vi "Strategy 5_Autotuning PID_With GUI - Copy (3).vi"() -> ()   [LabVIEW 2018]
doc: "This example demonstrates how to use the PID Design function to obtain PID parameters based on measured process."
uses:
  <vilib>/DAQmx/write.llb/DAQmx Write (Digital 1D Bool 1Chan 1Samp).vi
  <vilib>/Instr/_visa.llb/VISA Configure Serial Port (Instr).vi
  <vilib>/DAQmx/create/channels.llb/DAQmx Create Channel (DO-Digital Output).vi
  <vilib>/DAQmx/miscellaneous.llb/DAQmx Fill In Error Info.vi
  <vilib>/addons/control/pid/pid.llb/PID Advanced (DBL).vi
  <vilib>/addons/control/pid/autopid.llb/PID Autotuning Design (Ziegler-Nichols).vi
  <vilib>/addons/control/pid/autopid.llb/PID Autotuning Design (Cohen-Coon).vi
  <vilib>/addons/control/pid/autopid.llb/PID Autotuning Design (Chien-Hrones-Reswick).vi
  <vilib>/addons/control/pid/autopid.llb/PID Autotuning Design (Internal Model Control).vi
  <vilib>/addons/control/pid/NI_PID_autopid.lvlib
  <vilib>/addons/control/pid/NI_PID_pid.lvlib
  <vilib>/ptbypt/NI_PtbyPt.lvlib
panel:
  out "?":bool
  in  "Muscle Control":T1(tab)=enum."M-11"
  out "Tuned PID gains 12":T2={"proportional gain (Kc)"=1.9838195929127882, "integral time (Ti, min)"=0.01995856284686879, "derivative time (Td, min)"=0.0} {"derivative time (Td, min)" format="%#.6g"; "integral time (Ti, min)" format="%#.6g"; "proportional gain (Kc)" format="%#.6g"}
  in  "Accept gain 12":bool
  in  "Control 12":T3(tab)
  in  "Ziegler-Nichols speed 12":u16(ring) items=["Fast", "Normal", "Slow"]
  in  "Tuning specifications 12":u16(ring) items=["Regulator - 0 %", "Regulator -  20%", "Servo - 0%", "Servo - 20%"]
  in  "Multiplicative factor 12":dbl(slide)=1.0 scale=0.01..100.0
  in  "Type of controller 12":u16(ring)=2 items=["P", "PI", "PID"]
  in  "Stop 12":bool
  in  "PID Gains 12":T2={"proportional gain (Kc)"=0.1625, "integral time (Ti, min)"=1.25, "derivative time (Td, min)"=0.0} {"derivative time (Td, min)" format="%#.6g"; "integral time (Ti, min)" format="%#.6g"; "proportional gain (Kc)" format="%#.6g"}
  in  "Autotune 12":bool
  in  "Reinitialize 12":bool
  in  "Excitation 12":dbl=0.5 format="%.2f"
  in  "Automatic 12":bool=TRUE
  in  "MV: 12":dbl(slide)=20.39115328927357 scale=-100.0..100.0
  in  "Set Point 12":dbl(slide) scale=0.0..30.0
  out "PWM Output 12":bool
  out "Real time Data 12":dbl[][](graph)
  in  "Median sample length 21":i32=100
  in  "INLET 1 ON/OFF 3":bool=TRUE
  out "Tuned PID gains 11":T2={"proportional gain (Kc)"=1.9838195929127882, "integral time (Ti, min)"=0.01995856284686879, "derivative time (Td, min)"=0.0} {"derivative time (Td, min)" format="%#.6g"; "integral time (Ti, min)" format="%#.6g"; "proportional gain (Kc)" format="%#.6g"}
  in  "Accept gain 11":bool
  in  "Control 11":T3(tab)
  in  "Ziegler-Nichols speed 11":u16(ring) items=["Fast", "Normal", "Slow"]
  in  "Tuning specifications 11":u16(ring) items=["Regulator - 0 %", "Regulator -  20%", "Servo - 0%", "Servo - 20%"]
  in  "Multiplicative factor 11":dbl(slide)=1.0 scale=0.01..100.0
  in  "Type of controller 11":u16(ring)=2 items=["P", "PI", "PID"]
  in  "Excitation 11":dbl=0.5 format="%.2f"
  in  "Stop 11":bool
  in  "PID Gains 11":T2={"proportional gain (Kc)"=0.1625, "integral time (Ti, min)"=1.25, "derivative time (Td, min)"=0.0} {"derivative time (Td, min)" format="%#.6g"; "integral time (Ti, min)" format="%#.6g"; "proportional gain (Kc)" format="%#.6g"}
  in  "Autotune 11":bool
  in  "Reinitialize 11":bool
  in  "Automatic 11":bool=TRUE
  in  "MV: 11":dbl(slide)=20.39115328927357 scale=-100.0..100.0
  in  "Set Point 11":dbl(slide) scale=0.0..30.0
  out "PWM Output 11":bool
  out "Real time Data 11":dbl[][](graph)
  in  "Median sample length 20":i32=100
  in  "INLET 5 ON/OFF 3":bool=TRUE
  out "Tuned PID gains 10":T2={"proportional gain (Kc)"=1.9838195929127882, "integral time (Ti, min)"=0.01995856284686879, "derivative time (Td, min)"=0.0} {"derivative time (Td, min)" format="%#.6g"; "integral time (Ti, min)" format="%#.6g"; "proportional gain (Kc)" format="%#.6g"}
  in  "Accept gain 10":bool
  in  "Control 10":T3(tab)
  in  "Ziegler-Nichols speed 10":u16(ring) items=["Fast", "Normal", "Slow"]
  in  "Tuning specifications 10":u16(ring) items=["Regulator - 0 %", "Regulator -  20%", "Servo - 0%", "Servo - 20%"]
  in  "Multiplicative factor 10":dbl(slide)=1.0 scale=0.01..100.0
  in  "Type of controller 10":u16(ring)=2 items=["P", "PI", "PID"]
  in  "Stop 10":bool
  in  "PID Gains 10":T2={"proportional gain (Kc)"=0.1625, "integral time (Ti, min)"=1.25, "derivative time (Td, min)"=0.0} {"derivative time (Td, min)" format="%#.6g"; "integral time (Ti, min)" format="%#.6g"; "proportional gain (Kc)" format="%#.6g"}
  in  "Autotune 10":bool
  in  "Reinitialize 10":bool
  in  "Excitation 10":dbl=0.5 format="%.2f"
  in  "Automatic 10":bool=TRUE
  in  "MV: 10":dbl(slide)=20.39115328927357 scale=-100.0..100.0
  in  "Set Point 10":dbl(slide) scale=0.0..30.0
  out "PWM Output 10":bool
  out "Real time Data 10":dbl[][](graph)
  in  "Median sample length 19":i32=100
  in  "INLET 3 ON/OFF 3":bool=TRUE
  out "Tuned PID gains 9":T2={"proportional gain (Kc)"=1.9838195929127882, "integral time (Ti, min)"=0.01995856284686879, "derivative time (Td, min)"=0.0} {"derivative time (Td, min)" format="%#.6g"; "integral time (Ti, min)" format="%#.6g"; "proportional gain (Kc)" format="%#.6g"}
  in  "Accept gain 9":bool
  in  "Type of controller 9":u16(ring)=2 items=["P", "PI", "PID"]
  in  "Excitation 9":dbl=0.5 format="%.2f"
  in  "Control 9":T3(tab)
  in  "Ziegler-Nichols speed 9":u16(ring) items=["Fast", "Normal", "Slow"]
  in  "Tuning specifications 9":u16(ring) items=["Regulator - 0 %", "Regulator -  20%", "Servo - 0%", "Servo - 20%"]
  in  "Multiplicative factor 9":dbl(slide)=1.0 scale=0.01..100.0
  in  "Stop 9":bool
  in  "PID Gains 9":T2={"proportional gain (Kc)"=0.1625, "integral time (Ti, min)"=1.25, "derivative time (Td, min)"=0.0} {"derivative time (Td, min)" format="%#.6g"; "integral time (Ti, min)" format="%#.6g"; "proportional gain (Kc)" format="%#.6g"}
  in  "Autotune 9":bool
  in  "Reinitialize 9":bool
  in  "Automatic 9":bool=TRUE
  in  "MV: 9":dbl(slide)=20.39115328927357 scale=-100.0..100.0
  in  "Set Point 9":dbl(slide) scale=0.0..30.0
  out "PWM Output 9":bool
  out "Real time Data 9":dbl[][](graph)
  in  "Median sample length 18":i32=100
  in  "INLET 10 ON/OFF 2":bool=TRUE
  out "Tuned PID gains 8":T2={"proportional gain (Kc)"=1.9838195929127882, "integral time (Ti, min)"=0.01995856284686879, "derivative time (Td, min)"=0.0} {"derivative time (Td, min)" format="%#.6g"; "integral time (Ti, min)" format="%#.6g"; "proportional gain (Kc)" format="%#.6g"}
  in  "Accept gain 8":bool
  in  "Control 8":T3(tab)
  in  "Ziegler-Nichols speed 8":u16(ring) items=["Fast", "Normal", "Slow"]
  in  "Tuning specifications 8":u16(ring) items=["Regulator - 0 %", "Regulator -  20%", "Servo - 0%", "Servo - 20%"]
  in  "Multiplicative factor 8":dbl(slide)=1.0 scale=0.01..100.0
  in  "Type of controller 8":u16(ring)=2 items=["P", "PI", "PID"]
  in  "Stop 8":bool
  in  "PID Gains 8":T2={"proportional gain (Kc)"=0.1625, "integral time (Ti, min)"=1.25, "derivative time (Td, min)"=0.0} {"derivative time (Td, min)" format="%#.6g"; "integral time (Ti, min)" format="%#.6g"; "proportional gain (Kc)" format="%#.6g"}
  in  "Autotune 8":bool
  in  "Reinitialize 8":bool
  in  "Excitation 8":dbl=0.5 format="%.2f"
  in  "Automatic 8":bool=TRUE
  in  "MV: 8":dbl(slide)=20.39115328927357 scale=-100.0..100.0
  in  "Set Point 8":dbl(slide) scale=0.0..30.0
  out "PWM Output 8":bool
  out "Real time Data 8":dbl[][](graph)
  in  "Median sample length 17":i32=100
  in  "INLET 2 ON/OFF 2":bool=TRUE
  out "Tuned PID gains 7":T2={"proportional gain (Kc)"=1.9838195929127882, "integral time (Ti, min)"=0.01995856284686879, "derivative time (Td, min)"=0.0} {"derivative time (Td, min)" format="%#.6g"; "integral time (Ti, min)" format="%#.6g"; "proportional gain (Kc)" format="%#.6g"}
  in  "Accept gain 7":bool
  in  "Control 7":T3(tab)
  in  "Ziegler-Nichols speed 7":u16(ring) items=["Fast", "Normal", "Slow"]
  in  "Tuning specifications 7":u16(ring) items=["Regulator - 0 %", "Regulator -  20%", "Servo - 0%", "Servo - 20%"]
  in  "Multiplicative factor 7":dbl(slide)=1.0 scale=0.01..100.0
  in  "Type of controller 7":u16(ring)=2 items=["P", "PI", "PID"]
  in  "Stop 7":bool
  in  "PID Gains 7":T2={"proportional gain (Kc)"=0.1625, "integral time (Ti, min)"=1.25, "derivative time (Td, min)"=0.0} {"derivative time (Td, min)" format="%#.6g"; "integral time (Ti, min)" format="%#.6g"; "proportional gain (Kc)" format="%#.6g"}
  in  "Autotune 7":bool
  in  "Reinitialize 7":bool
  in  "Excitation 7":dbl=0.5 format="%.2f"
  in  "Automatic 7":bool=TRUE
  in  "MV: 7":dbl(slide)=20.39115328927357 scale=-100.0..100.0
  in  "Set Point 7":dbl(slide) scale=0.0..30.0
  out "PWM Output 7":bool
  out "Real time Data 7":dbl[][](graph)
  in  "Median sample length 16":i32=100
  in  "INLET 7 ON/OFF 2":bool=TRUE
  out "Tuned PID gains 6":T2={"proportional gain (Kc)"=1.9838195929127882, "integral time (Ti, min)"=0.01995856284686879, "derivative time (Td, min)"=0.0} {"derivative time (Td, min)" format="%#.6g"; "integral time (Ti, min)" format="%#.6g"; "proportional gain (Kc)" format="%#.6g"}
  in  "Accept gain 6":bool
  in  "Control 6":T3(tab)
  in  "Ziegler-Nichols speed 6":u16(ring) items=["Fast", "Normal", "Slow"]
  in  "Tuning specifications 6":u16(ring) items=["Regulator - 0 %", "Regulator -  20%", "Servo - 0%", "Servo - 20%"]
  in  "Multiplicative factor 6":dbl(slide)=1.0 scale=0.01..100.0
  in  "Type of controller 6":u16(ring)=2 items=["P", "PI", "PID"]
  in  "Stop 6":bool
  in  "PID Gains 6":T2={"proportional gain (Kc)"=0.1625, "integral time (Ti, min)"=1.25, "derivative time (Td, min)"=0.0} {"derivative time (Td, min)" format="%#.6g"; "integral time (Ti, min)" format="%#.6g"; "proportional gain (Kc)" format="%#.6g"}
  in  "Autotune 6":bool
  in  "Reinitialize 6":bool
  in  "Excitation 6":dbl=0.5 format="%.2f"
  in  "Automatic 6":bool=TRUE
  in  "MV: 6":dbl(slide)=20.39115328927357 scale=-100.0..100.0
  in  "Set Point 6":dbl(slide) scale=0.0..30.0
  out "PWM Output 6":bool
  out "Real time Data 6":dbl[][](graph)
  in  "Median sample length 15":i32=100
  in  "INLET 6 ON/OFF 2":bool=TRUE
  out "Tuned PID gains 5":T2={"proportional gain (Kc)"=1.9838195929127882, "integral time (Ti, min)"=0.01995856284686879, "derivative time (Td, min)"=0.0} {"derivative time (Td, min)" format="%#.6g"; "integral time (Ti, min)" format="%#.6g"; "proportional gain (Kc)" format="%#.6g"}
  in  "Accept gain 5":bool
  in  "Control 5":T3(tab)
  in  "Ziegler-Nichols speed 5":u16(ring) items=["Fast", "Normal", "Slow"]
  in  "Tuning specifications 5":u16(ring) items=["Regulator - 0 %", "Regulator -  20%", "Servo - 0%", "Servo - 20%"]
  in  "Multiplicative factor 5":dbl(slide)=1.0 scale=0.01..100.0
  in  "Type of controller 5":u16(ring)=2 items=["P", "PI", "PID"]
  in  "Stop 5":bool
  in  "PID Gains 5":T2={"proportional gain (Kc)"=0.1625, "integral time (Ti, min)"=1.25, "derivative time (Td, min)"=0.0} {"derivative time (Td, min)" format="%#.6g"; "integral time (Ti, min)" format="%#.6g"; "proportional gain (Kc)" format="%#.6g"}
  in  "Autotune 5":bool
  in  "Reinitialize 5":bool
  in  "Excitation 5":dbl=0.5 format="%.2f"
  in  "Automatic 5":bool=TRUE
  in  "MV: 5":dbl(slide)=20.39115328927357 scale=-100.0..100.0
  in  "Set Point 5":dbl(slide) scale=0.0..30.0
  out "PWM Output 5":bool
  out "Real time Data 5":dbl[][](graph)
  in  "Median sample length 14":i32=100
  in  "INLET 8 ON/OFF 2":bool=TRUE
  out "Tuned PID gains 4":T2={"proportional gain (Kc)"=1.9838195929127882, "integral time (Ti, min)"=0.01995856284686879, "derivative time (Td, min)"=0.0} {"derivative time (Td, min)" format="%#.6g"; "integral time (Ti, min)" format="%#.6g"; "proportional gain (Kc)" format="%#.6g"}
  in  "Accept gain 4":bool
  in  "Control 4":T3(tab)
  in  "Ziegler-Nichols speed 4":u16(ring) items=["Fast", "Normal", "Slow"]
  in  "Tuning specifications 4":u16(ring) items=["Regulator - 0 %", "Regulator -  20%", "Servo - 0%", "Servo - 20%"]
  in  "Multiplicative factor 4":dbl(slide)=1.0 scale=0.01..100.0
  in  "Type of controller 4":u16(ring)=2 items=["P", "PI", "PID"]
  in  "Stop 4":bool
  in  "PID Gains 4":T2={"proportional gain (Kc)"=0.1625, "integral time (Ti, min)"=1.25, "derivative time (Td, min)"=0.0} {"derivative time (Td, min)" format="%#.6g"; "integral time (Ti, min)" format="%#.6g"; "proportional gain (Kc)" format="%#.6g"}
  in  "Autotune 4":bool
  in  "Reinitialize 4":bool
  in  "Excitation 4":dbl=0.5 format="%.2f"
  in  "Automatic 4":bool=TRUE
  in  "MV: 4":dbl(slide)=20.39115328927357 scale=-100.0..100.0
  in  "Set Point 4":dbl(slide) scale=0.0..30.0
  out "PWM Output 4":bool
  out "Real time Data 4":dbl[][](graph)
  in  "Median sample length 9":i32=100
  in  "INLET 9 ON/OFF 2":bool=TRUE
  out "Tuned PID gains 3":T2={"proportional gain (Kc)"=1.9838195929127882, "integral time (Ti, min)"=0.01995856284686879, "derivative time (Td, min)"=0.0} {"derivative time (Td, min)" format="%#.6g"; "integral time (Ti, min)" format="%#.6g"; "proportional gain (Kc)" format="%#.6g"}
  in  "Accept gain 3":bool
  in  "Control 3":T3(tab)
  in  "Ziegler-Nichols speed 3":u16(ring) items=["Fast", "Normal", "Slow"]
  in  "Tuning specifications 3":u16(ring) items=["Regulator - 0 %", "Regulator -  20%", "Servo - 0%", "Servo - 20%"]
  in  "Multiplicative factor 3":dbl(slide)=1.0 scale=0.01..100.0
  in  "Type of controller 3":u16(ring)=2 items=["P", "PI", "PID"]
  in  "Stop 3":bool
  in  "PID Gains 3":T2={"proportional gain (Kc)"=0.1625, "integral time (Ti, min)"=1.25, "derivative time (Td, min)"=0.0} {"derivative time (Td, min)" format="%#.6g"; "integral time (Ti, min)" format="%#.6g"; "proportional gain (Kc)" format="%#.6g"}
  in  "Autotune 3":bool
  in  "Reinitialize 3":bool
  in  "Excitation 3":dbl=0.5 format="%.2f"
  in  "Automatic 3":bool=TRUE
  in  "MV: 3":dbl(slide)=20.39115328927357 scale=-100.0..100.0
  in  "Set Point 3":dbl(slide) scale=0.0..30.0
  out "PWM Output 3":bool
  out "Real time Data 3":dbl[][](graph)
  in  "Median sample length 13":i32=100
  in  "INLET 10 ON/OFF":bool=TRUE
  in  "INLET":bool=TRUE
  out "PWM Output":bool
  out "Real time Data":dbl[][](graph)
  in  "MV:":dbl(slide)=20.39115328927357 scale=-100.0..100.0
  in  "Set Point":dbl(slide) scale=0.0..30.0
  in  "Median sample length":i32=100
  in  "Excitation":dbl=0.5 format="%.2f"
  in  "Type of controller":u16(ring)=2 items=["P", "PI", "PID"]
  in  "Control":T3(tab)
  in  "Ziegler-Nichols speed":u16(ring) items=["Fast", "Normal", "Slow"]
  in  "Tuning specifications":u16(ring) items=["Regulator - 0 %", "Regulator -  20%", "Servo - 0%", "Servo - 20%"]
  in  "Multiplicative factor":dbl(slide)=1.0 scale=0.01..100.0
  in  "Automatic":bool=TRUE
  in  "Reinitialize":bool
  in  "Accept gain":bool
  out "Tuned PID gains":T2={"proportional gain (Kc)"=1.9838195929127882, "integral time (Ti, min)"=0.01995856284686879, "derivative time (Td, min)"=0.0} {"derivative time (Td, min)" format="%#.6g"; "integral time (Ti, min)" format="%#.6g"; "proportional gain (Kc)" format="%#.6g"}
  in  "Autotune":bool
  in  "PID Gains":T2={"proportional gain (Kc)"=0.1625, "integral time (Ti, min)"=1.25, "derivative time (Td, min)"=0.0} {"derivative time (Td, min)" format="%#.6g"; "integral time (Ti, min)" format="%#.6g"; "proportional gain (Kc)" format="%#.6g"}
  in  "Stop":bool
  out "Tuned PID gains 2":T2={"proportional gain (Kc)"=1.9838195929127882, "integral time (Ti, min)"=0.01995856284686879, "derivative time (Td, min)"=0.0} {"derivative time (Td, min)" format="%#.6g"; "integral time (Ti, min)" format="%#.6g"; "proportional gain (Kc)" format="%#.6g"}
  in  "Accept gain 2":bool
  in  "Control 2":T3(tab)
  in  "Ziegler-Nichols speed 2":u16(ring) items=["Fast", "Normal", "Slow"]
  in  "Tuning specifications 2":u16(ring) items=["Regulator - 0 %", "Regulator -  20%", "Servo - 0%", "Servo - 20%"]
  in  "Multiplicative factor 2":dbl(slide)=1.0 scale=0.01..100.0
  in  "Type of controller 2":u16(ring)=2 items=["P", "PI", "PID"]
  in  "Stop 2":bool
  in  "PID Gains 2":T2={"proportional gain (Kc)"=0.1625, "integral time (Ti, min)"=1.25, "derivative time (Td, min)"=0.0} {"derivative time (Td, min)" format="%#.6g"; "integral time (Ti, min)" format="%#.6g"; "proportional gain (Kc)" format="%#.6g"}
  in  "Autotune 2":bool
  in  "Reinitialize 2":bool
  in  "Excitation 2":dbl=0.5 format="%.2f"
  in  "Automatic 2":bool=TRUE
  in  "MV: 2":dbl(slide)=20.39115328927357 scale=-100.0..100.0
  in  "Set Point 2":dbl(slide) scale=0.0..30.0
  out "PWM Output 2":bool
  out "Real time Data 2":dbl[][](graph)
  in  "Median sample length 12":i32=100
  in  "INLET 12 ON/OFF":bool=TRUE
  in  "M-11":i32=5
  in  "M-12":i32=5
  in  "M-10":i32=5
  in  "M-9":i32=5
  in  "M-8":i32=5
  in  "M-6":i32=5
  in  "M-7":i32=5
  in  "M-2":i32=5
  in  "M-4":i32=5
  in  "M-3":i32=5
  in  "M-5":i32=5
  in  "M-1":i32=5
  out "Identified Plant Parameters":T4={"Plant Gain (K)"=1.7609511324977591, "Time Constant (T)"=1.9621978490901302, "Dead Time (L)"=0.22467425343567116}
  out "Control Output":dbl[](graph)
  out "Measurement":dbl[](graph)
  out "Stimulus operating point":dbl=20.314221540357543
  out "Response operating point":dbl=51.08345461694337
  out "Stimulus operating point 2":dbl=20.314221540357543
  out "Response operating point 2":dbl=51.08345461694337
  out "Identified Plant Parameters 2":T4={"Plant Gain (K)"=1.7609511324977591, "Time Constant (T)"=1.9621978490901302, "Dead Time (L)"=0.22467425343567116}
  out "Control Output 2":dbl[](graph)
  out "Measurement 2":dbl[](graph)
  out "Stimulus operating point 3":dbl=20.314221540357543
  out "Response operating point 3":dbl=51.08345461694337
  out "Identified Plant Parameters 3":T4={"Plant Gain (K)"=1.7609511324977591, "Time Constant (T)"=1.9621978490901302, "Dead Time (L)"=0.22467425343567116}
  out "Control Output 3":dbl[](graph)
  out "Measurement 3":dbl[](graph)
  out "Stimulus operating point 4":dbl=20.314221540357543
  out "Response operating point 4":dbl=51.08345461694337
  out "Identified Plant Parameters 4":T4={"Plant Gain (K)"=1.7609511324977591, "Time Constant (T)"=1.9621978490901302, "Dead Time (L)"=0.22467425343567116}
  out "Control Output 4":dbl[](graph)
  out "Measurement 4":dbl[](graph)
  out "Stimulus operating point 5":dbl=20.314221540357543
  out "Response operating point 5":dbl=51.08345461694337
  out "Identified Plant Parameters 5":T4={"Plant Gain (K)"=1.7609511324977591, "Time Constant (T)"=1.9621978490901302, "Dead Time (L)"=0.22467425343567116}
  out "Control Output 5":dbl[](graph)
  out "Measurement 5":dbl[](graph)
  out "Stimulus operating point 6":dbl=20.314221540357543
  out "Response operating point 6":dbl=51.08345461694337
  out "Identified Plant Parameters 6":T4={"Plant Gain (K)"=1.7609511324977591, "Time Constant (T)"=1.9621978490901302, "Dead Time (L)"=0.22467425343567116}
  out "Control Output 6":dbl[](graph)
  out "Measurement 6":dbl[](graph)
  out "Stimulus operating point 7":dbl=20.314221540357543
  out "Response operating point 7":dbl=51.08345461694337
  out "Identified Plant Parameters 7":T4={"Plant Gain (K)"=1.7609511324977591, "Time Constant (T)"=1.9621978490901302, "Dead Time (L)"=0.22467425343567116}
  out "Control Output 7":dbl[](graph)
  out "Measurement 7":dbl[](graph)
  out "Stimulus operating point 8":dbl=20.314221540357543
  out "Response operating point 8":dbl=51.08345461694337
  out "Identified Plant Parameters 8":T4={"Plant Gain (K)"=1.7609511324977591, "Time Constant (T)"=1.9621978490901302, "Dead Time (L)"=0.22467425343567116}
  out "Control Output 8":dbl[](graph)
  out "Measurement 8":dbl[](graph)
  out "Stimulus operating point 9":dbl=20.314221540357543
  out "Response operating point 9":dbl=51.08345461694337
  out "Identified Plant Parameters 9":T4={"Plant Gain (K)"=1.7609511324977591, "Time Constant (T)"=1.9621978490901302, "Dead Time (L)"=0.22467425343567116}
  out "Control Output 9":dbl[](graph)
  out "Measurement 9":dbl[](graph)
  out "Stimulus operating point 10":dbl=20.314221540357543
  out "Response operating point 10":dbl=51.08345461694337
  out "Identified Plant Parameters 10":T4={"Plant Gain (K)"=1.7609511324977591, "Time Constant (T)"=1.9621978490901302, "Dead Time (L)"=0.22467425343567116}
  out "Control Output 10":dbl[](graph)
  out "Measurement 10":dbl[](graph)
  out "Stimulus operating point 11":dbl=20.314221540357543
  out "Response operating point 11":dbl=51.08345461694337
  out "Identified Plant Parameters 11":T4={"Plant Gain (K)"=1.7609511324977591, "Time Constant (T)"=1.9621978490901302, "Dead Time (L)"=0.22467425343567116}
  out "Control Output 11":dbl[](graph)
  out "Measurement 11":dbl[](graph)
  out "Stimulus operating point 12":dbl=20.314221540357543
  out "Response operating point 12":dbl=51.08345461694337
  out "Identified Plant Parameters 12":T4={"Plant Gain (K)"=1.7609511324977591, "Time Constant (T)"=1.9621978490901302, "Dead Time (L)"=0.22467425343567116}
  out "Control Output 12":dbl[](graph)
  out "Measurement 12":dbl[](graph)
  in  "XYZAER":T5(array[cluster]) {"r" format="%1_6f"; "e" format="%1_6f"; "a" format="%1_6f"; "z" format="%1_6f"; "y" format="%1_6f"; "x" format="%1_6f"}
  out "Connected":bool
  out "Start Time Text":string
  out "Stop Time Text":string
  out "Elapsed Time Text":string
  out "HostFrameCount":u32
  out "Running":bool
  out "Loop Iter":i32
  out "PnoData":bool
  in  "stop":bool
  out "error out":errorcluster {"code" format="%.0x"}
  out "Position Sensor Data":cluster{dbl, "x":sgl}[](graph)
  out "Sensor Raw Value 2":i32
  in  "COM Port-Sensor 2":refnum<visa-resource-name>="COM5"
  in  "upper/lower infle":enum32{"Page 1", "Page 2"}(tab)
  out "Force in Kilograms":dbl(graph)
  out "Force in Newtons":dbl(graph)
  in  "lower/upper infle":enum32{"Page 1", "Page 2"}(tab)
  out "Force in Newtons 2":dbl(graph)
  out "Force in Kilograms 2":dbl(graph)
  in  "COM Port-Sensor 1":refnum<visa-resource-name>="COM4"
  out "Sensor Raw Value":i32
  in  "Tab Control":T6(tab)
  in  "Instructions":string="Overview: This example demonstrates how to use the PID Autotuning Design to obtain PID parameters based on setpoint and process variable collected in another loop.\nInstructions:\n1. Run the VI and wait until the process variable (PV) reaches near setpoint (SP).\n2.  In the PID Autotuning Design section, select the type of algorithm, type of controller and excitation amplitude for the 'open loop step response'. Then, click Autotune to start the process. Select the Identified Plant Parameter tab and see the results from the identification.\n3.  When the tuned PID gains do not change anymore, the identification is done and you have the option to accept by clicking Accept gain, which will transfer the new gain to PID Gains.\n4. Click the Autotune button again to go back to the automatic control state. You can try different options and repeat this process.\n5. Click Stop to stop the VI.\n"
  in  "Instructions 2":string="Overview: This example demonstrates how to use the PID Autotuning Design to obtain PID parameters based on setpoint and process variable collected in another loop.\nInstructions:\n1. Run the VI and wait until the process variable (PV) reaches near setpoint (SP).\n2.  In the PID Autotuning Design section, select the type of algorithm, type of controller and excitation amplitude for the 'open loop step response'. Then, click Autotune to start the process. Select the Identified Plant Parameter tab and see the results from the identification.\n3.  When the tuned PID gains do not change anymore, the identification is done and you have the option to accept by clicking Accept gain, which will transfer the new gain to PID Gains.\n4. Click the Autotune button again to go back to the automatic control state. You can try different options and repeat this process.\n5. Click Stop to stop the VI.\n"
  in  "Instructions 3":string="Overview: This example demonstrates how to use the PID Autotuning Design to obtain PID parameters based on setpoint and process variable collected in another loop.\nInstructions:\n1. Run the VI and wait until the process variable (PV) reaches near setpoint (SP).\n2.  In the PID Autotuning Design section, select the type of algorithm, type of controller and excitation amplitude for the 'open loop step response'. Then, click Autotune to start the process. Select the Identified Plant Parameter tab and see the results from the identification.\n3.  When the tuned PID gains do not change anymore, the identification is done and you have the option to accept by clicking Accept gain, which will transfer the new gain to PID Gains.\n4. Click the Autotune button again to go back to the automatic control state. You can try different options and repeat this process.\n5. Click Stop to stop the VI.\n"
  # "Pressure Alarm"
  # "Position Sensor Data"
  # "Force Sensor Data"
  # "PID Controller"
  # "PID Autotuning Design"
  # "No additional parameters"
  # "PID Controller"
  # "PID Autotuning Design"
  # "No additional parameters"
  # "PID Controller"
  # "PID Autotuning Design"
  # "No additional parameters"
  # "PID Controller"
  # "PID Autotuning Design"
  # "No additional parameters"
  # "PID Controller"
  # "PID Autotuning Design"
  # "No additional parameters"
  # "PID Controller"
  # "PID Autotuning Design"
  # "No additional parameters"
  # "PID Controller"
  # "PID Autotuning Design"
  # "No additional parameters"
  # "Muscle Control"
  # "PID Controller"
  # "PID Autotuning Design"
  # "No additional parameters"
  # "PID Controller"
  # "PID Autotuning Design"
  # "No additional parameters"
  # "PID Controller"
  # "PID Autotuning Design"
  # "No additional parameters"
  # "Muscle Control"
  # "PID Controller"
  # "PID Autotuning Design"
  # "No additional parameters"
  # "PID Controller"
  # "PID Autotuning Design"
  # "No additional parameters"
  # "Pressure Cut Off to trigger the alarm"
  # "M-11"
  # "M-12"
  # "M-10"
  # "M-9"
  # "M-8"
  # "M-6"
  # "M-7"
  # "M-2"
  # "M-4"
  # "M-3"
  # "M-5"
  # "M-1"
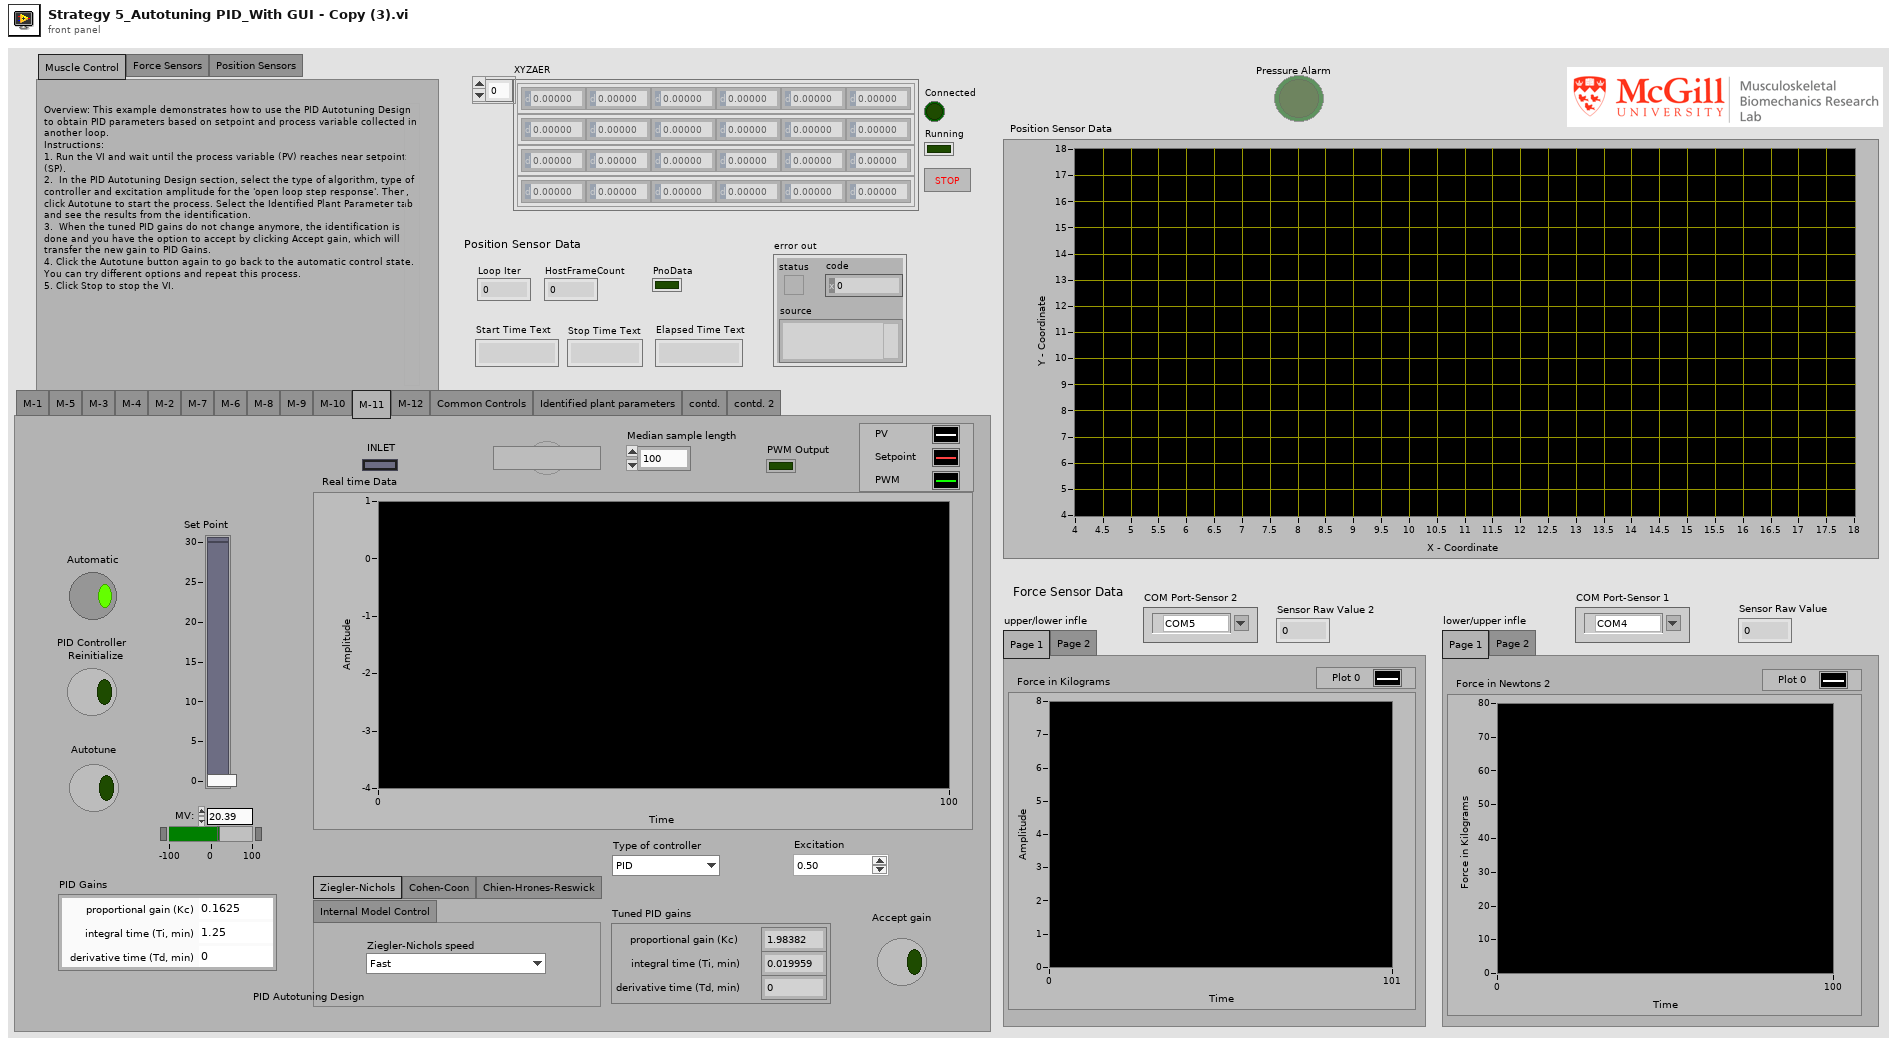
[diagram p1: front panel]
types:
  T1 = enum32{"M-1", "M-5", "M-3", "M-4", "M-2", "M-7", "M-6", "M-8", "M-9", "M-10", "M-11", "M-12", "Common Controls", "Identified plant parameters", "contd.", "contd. 2"}
  T2 = cluster{"proportional gain (Kc)":dbl, "integral time (Ti, min)":dbl, "derivative time (Td, min)":dbl}
  T3 = enum32{"Ziegler-Nichols", "Cohen-Coon", "Chien-Hrones-Reswick", "Internal Model Control"}
  T4 = cluster{"Plant Gain (K)":dbl, "Time Constant (T)":dbl, "Dead Time (L)":dbl}
  T5 = cluster{"x":sgl, "y":sgl, "z":sgl, "a":sgl, "e":sgl, "r":sgl}[]
  T6 = enum32{"Muscle Control", "Force Sensors", "Position Sensors"}
  T7 = cluster{"static gain":dbl, "lag (s)":dbl, "deadtime (s)":dbl, "load":dbl, "deadband":dbl, "sensor noise":dbl, "initial PV":dbl, "plant noise":dbl}
  T8 = cluster{"x":sgl, "y":sgl, "z":sgl, "a":sgl, "e":sgl, "r":sgl}
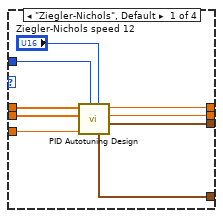
[diagram p2: hidden frame]
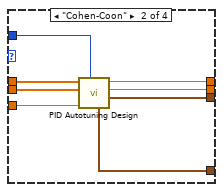
[diagram p3: hidden frame]
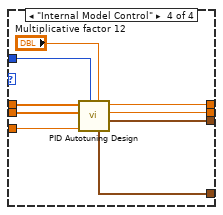
[diagram p4: hidden frame]
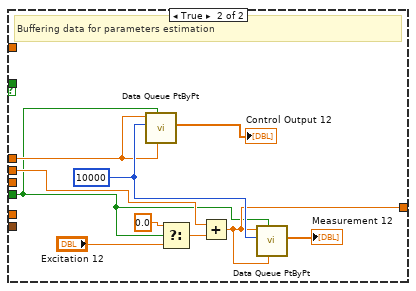
[diagram p6: hidden frame]
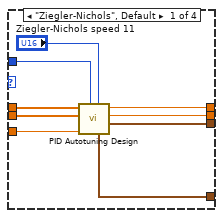
[diagram p7: hidden frame]
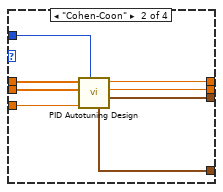
[diagram p8: hidden frame]
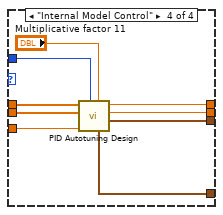
[diagram p9: hidden frame]
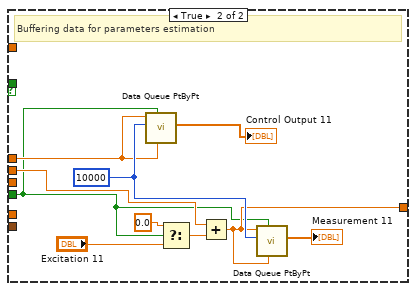
[diagram p11: hidden frame]
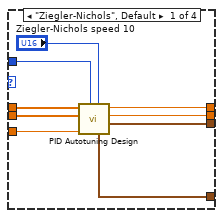
[diagram p12: hidden frame]
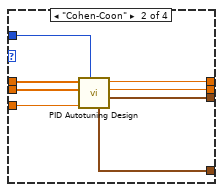
[diagram p13: hidden frame]
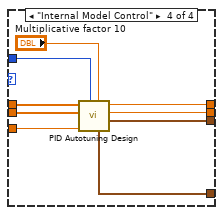
[diagram p14: hidden frame]
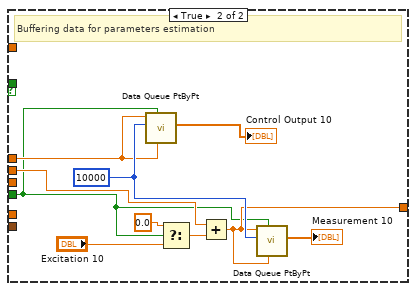
[diagram p16: hidden frame]
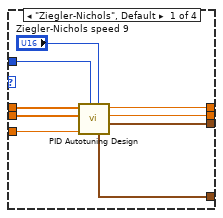
[diagram p17: hidden frame]
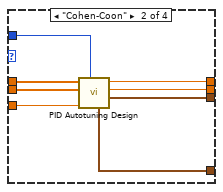
[diagram p18: hidden frame]
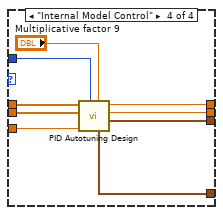
[diagram p19: hidden frame]
diagram:
  w16 = 0.0 ("output")
  w19 = FALSE ("Stop")
  w22 = 0.0 ("output")
  w25 = FALSE ("Stop")
  w28 = 0.0 ("output")
  w31 = FALSE ("Stop")
  w34 = 0.0 ("output")
  w37 = FALSE ("Stop")
  w40 = 0.0 ("output")
  w43 = FALSE ("Stop")
  w46 = 0.0 ("output")
  w49 = FALSE ("Stop")
  w52 = 0.0 ("output")
  w55 = FALSE ("Stop")
  w58 = 0.0 ("output")
  w61 = FALSE ("Stop")
  w64 = 0.0 ("output")
  w67 = FALSE ("Stop")
  w70 = 0.0 ("output")
  w73 = FALSE ("Stop")
  w76 = 0.0 ("output")
  w79 = FALSE ("Stop")
  w84 = 2400  # BufferFrameCount
  w118 = 0.0 ("output")
  w121 = FALSE ("Stop")
  # "Muscle-1 PID CONTROL LOOP (Auto Tuning)"
  # "Muscle-5 PID CONTROL LOOP (Auto Tuning)"
  # "Muscle-3 PID CONTROL LOOP (Auto Tuning)"
  # "Muscle-4 PID CONTROL LOOP (Auto Tuning)"
  # "Muscle-2 PID CONTROL LOOP (Auto Tuning)"
  # "Muscle-7 PID CONTROL LOOP (Auto Tuning)"
  # "Muscle-6 PID CONTROL LOOP (Auto Tuning)"
  # "Muscle-8 PID CONTROL LOOP (Auto Tuning)"
  # "Muscle-9 PID CONTROL LOOP (Auto Tuning)"
  # "Muscle-10 PID CONTROL LOOP (Auto Tuning)"
  # "Muscle-12 PID CONTROL LOOP (Auto Tuning)"
  # "Muscle-11 PID CONTROL LOOP (Auto Tuning)"
  # "FORCE SENSOR CONTROL LOOP"
  # "POSITION SENSOR CONTROL LOOP"
  # "Pressure Alarm"
  # "8. Close Tracker connection."
  # "3. Query Max num sensors supported by the tracker."
  # "4. Allocate raw buffer to hold 2400 frames of data."
  # "5. Start Continuous mode."
  # "7. Stop Continuous mode."
  # "6. Start the loop. Loop exits when Stop Button is hit."
  n1 = call "DAQ Assistant"() -> ("data"=w14:dynamicdata)  [unwired: 17 in, 2 out]
  n2 = while {
    shift-left: 0.0 ("Plant Output") -> [w188]
    shift-right: [w183] -> _
    tunnel: w55 -> [_]
    shift-right: [w169] -> _
    shift-left: 0.01 -> [w167]
    shift-right: [w141] -> _
    shift-left: TRUE -> [w166]
    shift-right: [w143] -> _
    shift-left: w52 -> [w165]
    shift-right: [w168] -> _
    shift-left: w52 -> [w164]
    tunnel: [w138] -> w51
    tunnel: w14 -> [w124]
    tunnel: [w123] -> w7
    stop <- "Stop 6" stop-if-true
    w129 = 1 items=["one channel for each line", "one channel for all lines"] ("line grouping")
    w138 = 0.05 ("Sampling Time dt (s)")
    w147 = 1 items=["one channel for each line", "one channel for all lines"] ("line grouping")
    w155 = 0.5 ("x")
    w182 = T7 {"static gain"=2.5, "lag (s)"=2.5, "deadtime (s)"=0.01, "load"=0.0, "deadband"=0.0, "sensor noise"=0.0, "initial PV"=30.0, "plant noise"=0.0}  # Process parameters
    w184 = FALSE  # Integrator ?
    # "C."
    # "Inlet 11"
    # "Exhaust 6"
    # "B."
    # "A."
    # "A.Output to PWM Logic \nB. Simulated Plant\nC. Draw Chart"
    # "Main PID Loop Control"
    n3 = Multiply(x=w138, y=1000.0) -> (x*y=w181:dbl)
    n4 = Not(x="Autotune 6") -> (.not. x?=w185:bool)
    n5 = feedback #1() -> (w190:bool)  [unwired: 1 in]
    n6 = feedback-in #1("Autotune 6") -> ()
    n7 = Wait Until Next ms Multiple(millisecond multiple=w181) -> ()  [unwired: 1 out]
    n8 = Exclusive Or(1:w190, 2:"Autotune 6") -> (0:w189:bool)
    n9 = feedback #2() -> (w187:dbl)  [unwired: 1 in]
    n10 = Multiply(x=w124, y=-1000.0) -> (x*y=w171:dynamicdata)
    n11 = call <vilib>:"Median PtByPt.vi"("sample length"="Median sample length 15", "x"=w171) -> ("median"=w170:dbl)  [unwired: 2 in, 1 out]
    n12 = Square(x=w170) -> (x^2=w178:dbl)
    n13 = Multiply(x=w170, y=-39.646) -> (x*y=w174:dbl)
    n14 = Multiply(x=w178, y=0.2324) -> (x*y=w175:dbl)
    n15 = Add(x=w174, y=w175) -> (x+y=w173:dbl)
    n16 = Add(x=1678.0, y=w173) -> (x+y=w136:dbl)
    n17 = case shown="False" "Autotune 6" {
      tunnel: w138 -> [w205 _]
      tunnel: [w194 w210] -> w143
      tunnel: w188 -> [_ w209]
      tunnel: "PID Gains 6" -> [w204 _]
      tunnel: "Reinitialize 6" -> [w201 _]
      tunnel: w189 -> [w203 w208]
      tunnel: w187 -> [_ w212]
      tunnel: w136 -> [w197 _]
      tunnel: "Set Point 6" -> [w196 _]
      frame False {
        # "This code is to have 'bumpless' transfer from autotuning"
        n18 = Not(x=w203) -> (.not. x?=w200:bool)
        n19 = And(x="Automatic 6", y=w200) -> (x .and. y?=w202:bool)
        n20 = call-poly <vilib>:"PID Advanced.vi"("setpoint"=w196, "auto? (T)"=w202, "manual control"="MV: 6", "process variable"=w197, "alpha"=10.0, "PID gains"=w204, "dt (s)"=w205, "reinitialize? (F)"=w201) -> ("output"=w194:dbl)  [unwired: 6 in, 1 out]
      }
      frame True {
        w215 = 10000 ("sample length")
        # "Buffering data for parameters estimation"
        n21 = call <vilib>:"Data Queue PtByPt.vi"("initial queue element"=w209, "initialize"=w208, "sample length"=w215, "input data point"=w209) -> ("Current Queue"=→"Control Output 6":dbl[])  [unwired: 3 in, 4 out]
        n22 = Select(t=0.0, s=w208, f="Excitation 6") -> (s? t:f=w213:dbl)
        n23 = Add(x=w212, y=w213) -> (x+y=w210:dbl)
        n24 = call <vilib>:"Data Queue PtByPt.vi"("initial queue element"=w210, "initialize"=w208, "sample length"=w215, "input data point"=w210) -> ("Current Queue"=→"Measurement 6":dbl[])  [unwired: 3 in, 4 out]
      }
    }
    n25 = feedback-in #2(w143, w185) -> ()
    n26 = Greater?(x=w136, y="M-6") -> (0:w123:bool)
    n27 = Add(x=w167, y=w155) -> (x+y=w156:dbl)
    n28 = Subtract(x=w167, y=w155) -> (x-y=w154:dbl)
    n29 = Equal?(x=w165, y=w143) -> (x = y?=w162:bool)
    n30 = Greater?(x=w143, y=w165) -> (0:w161:bool)
    n31 = Select(t=w166, s=w162, f=w161) -> (s? t:f=w141:bool)
    "PWM Output 6" <- w141
    n32 = call "Plant System.vi"("Integrator ?"=w184, "Plant Input"=w143, "dt (s)"=w138, "process parameters"=w182) -> ("Plant Output"=w183:dbl)  [unwired: 11 in]
    n33 = Increment(x="Set Point 6") -> (x+1=w160:dbl)
    n34 = Decrement(x="Set Point 6") -> (x-1=w159:dbl)
    n35 = Select(t=w156, s=w141, f=w154) -> (s? t:f=w169:dbl)
    n36 = Select(t=w160, s=w141, f=w159) -> (s? t:f=w158:dbl)
    n37 = Not(x=w141) -> (.not. x?=w140:bool)
    n38 = call-poly <vilib>:"DAQmx Create Virtual Channel.vi"("lines"=tag "cDAQ1Mod1/port0/line4", "line grouping"=w147) -> ("task out"=w149:refnum<k21>, "error out"=w148:errorcluster)  [unwired: 12 in]
    n39 = call-poly <vilib>:"DAQmx Create Virtual Channel.vi"("lines"=tag "cDAQ1Mod2/port0/line4", "line grouping"=w129) -> ("task out"=w131:refnum<k21>, "error out"=w130:errorcluster)  [unwired: 12 in]
    n40 = Build Array(w136, "Set Point 6", w158) -> (w157:dbl[])
    n41 = Initialize Array("INLET 6 ON/OFF 2", 1 ("dimension size")) -> (w126:bool[])
    n42 = Initialize Array(w140, 1 ("dimension size")) -> (w144:bool[])
    n43 = local write "MV: 6"(w143) -> ()
    n44 = Add(x=w164, y=w167) -> (x+y=w168:dbl)
    n45 = Build Array(w157) -> (→"Real time Data 6":dbl[][])
    n46 = call-poly <vilib>:"DAQmx Write.vi"("task/channels in"=w149, "auto start"=TRUE, "data"=w144, "error in"=w148) -> ("task out"=w151:refnum<k21>, "error out"=w152:errorcluster)  [unwired: 9 in, 1 out]
    n47 = call-poly <vilib>:"DAQmx Write.vi"("task/channels in"=w131, "auto start"=TRUE, "data"=w126, "error in"=w130) -> ("task out"=w133:refnum<k21>, "error out"=w134:errorcluster)  [unwired: 9 in, 1 out]
    n48 = call <vilib>:"DAQmx Clear Task.vi"("task in"=w151, "error in"=w152) -> ("error out"=w146:errorcluster)  [unwired: 13 in]
    n49 = call <vilib>:"DAQmx Clear Task.vi"("task in"=w133, "error in"=w134) -> ("error out"=w128:errorcluster)  [unwired: 13 in]
    n50 = call <vilib>:"Simple Error Handler.vi"("error in (no error)"=w146) -> ()  [unwired: 4 in, 5 out]
    n51 = call <vilib>:"Simple Error Handler.vi"("error in (no error)"=w128) -> ()  [unwired: 4 in, 5 out]
  }
  n52 = while {
    shift-left: 0.0 ("Plant Output") -> [w281]
    shift-right: [w276] -> _
    tunnel: w67 -> [_]
    shift-right: [w262] -> _
    shift-left: 0.01 -> [w260]
    shift-right: [w234] -> _
    shift-left: TRUE -> [w259]
    shift-right: [w236] -> _
    shift-left: w64 -> [w258]
    shift-right: [w261] -> _
    shift-left: w64 -> [w257]
    tunnel: [w231] -> w63
    tunnel: w14 -> [w217]
    tunnel: [w216] -> w9
    stop <- "Stop 4" stop-if-true
    w222 = 1 items=["one channel for each line", "one channel for all lines"] ("line grouping")
    w231 = 0.05 ("Sampling Time dt (s)")
    w240 = 1 items=["one channel for each line", "one channel for all lines"] ("line grouping")
    w248 = 0.5 ("x")
    w275 = T7 {"static gain"=2.5, "lag (s)"=2.5, "deadtime (s)"=0.01, "load"=0.0, "deadband"=0.0, "sensor noise"=0.0, "initial PV"=30.0, "plant noise"=0.0}  # Process parameters
    w277 = FALSE  # Integrator ?
    # "C."
    # "Inlet 11"
    # "Exhaust 9"
    # "B."
    # "A."
    # "A.Output to PWM Logic \nB. Simulated Plant\nC. Draw Chart"
    # "Main PID Loop Control"
    n53 = Multiply(x=w231, y=1000.0) -> (x*y=w274:dbl)
    n54 = Not(x="Autotune 4") -> (.not. x?=w278:bool)
    n55 = feedback #3() -> (w283:bool)  [unwired: 1 in]
    n56 = feedback-in #3("Autotune 4") -> ()
    n57 = Wait Until Next ms Multiple(millisecond multiple=w274) -> ()  [unwired: 1 out]
    n58 = Exclusive Or(1:w283, 2:"Autotune 4") -> (0:w282:bool)
    n59 = feedback #4() -> (w280:dbl)  [unwired: 1 in]
    n60 = Multiply(x=w217, y=-1000.0) -> (x*y=w264:dynamicdata)
    n61 = call <vilib>:"Median PtByPt.vi"("sample length"="Median sample length 9", "x"=w264) -> ("median"=w263:dbl)  [unwired: 2 in, 1 out]
    n62 = Square(x=w263) -> (x^2=w271:dbl)
    n63 = Multiply(x=w263, y=-39.646) -> (x*y=w267:dbl)
    n64 = Multiply(x=w271, y=0.2324) -> (x*y=w268:dbl)
    n65 = Add(x=w267, y=w268) -> (x+y=w266:dbl)
    n66 = Add(x=1678.0, y=w266) -> (x+y=w229:dbl)
    n67 = case shown="False" "Autotune 4" {
      tunnel: w231 -> [w298 _]
      tunnel: [w287 w303] -> w236
      tunnel: w281 -> [_ w302]
      tunnel: "PID Gains 4" -> [w297 _]
      tunnel: "Reinitialize 4" -> [w294 _]
      tunnel: w282 -> [w296 w301]
      tunnel: w280 -> [_ w305]
      tunnel: w229 -> [w290 _]
      tunnel: "Set Point 4" -> [w289 _]
      frame False {
        # "This code is to have 'bumpless' transfer from autotuning"
        n68 = Not(x=w296) -> (.not. x?=w293:bool)
        n69 = And(x="Automatic 4", y=w293) -> (x .and. y?=w295:bool)
        n70 = call-poly <vilib>:"PID Advanced.vi"("setpoint"=w289, "auto? (T)"=w295, "manual control"="MV: 4", "process variable"=w290, "alpha"=10.0, "PID gains"=w297, "dt (s)"=w298, "reinitialize? (F)"=w294) -> ("output"=w287:dbl)  [unwired: 6 in, 1 out]
      }
      frame True {
        w308 = 10000 ("sample length")
        # "Buffering data for parameters estimation"
        n71 = call <vilib>:"Data Queue PtByPt.vi"("initial queue element"=w302, "initialize"=w301, "sample length"=w308, "input data point"=w302) -> ("Current Queue"=→"Control Output 4":dbl[])  [unwired: 3 in, 4 out]
        n72 = Select(t=0.0, s=w301, f="Excitation 4") -> (s? t:f=w306:dbl)
        n73 = Add(x=w305, y=w306) -> (x+y=w303:dbl)
        n74 = call <vilib>:"Data Queue PtByPt.vi"("initial queue element"=w303, "initialize"=w301, "sample length"=w308, "input data point"=w303) -> ("Current Queue"=→"Measurement 4":dbl[])  [unwired: 3 in, 4 out]
      }
    }
    n75 = feedback-in #4(w236, w278) -> ()
    n76 = Greater?(x=w229, y="M-9") -> (0:w216:bool)
    n77 = Add(x=w260, y=w248) -> (x+y=w249:dbl)
    n78 = Subtract(x=w260, y=w248) -> (x-y=w247:dbl)
    n79 = Equal?(x=w258, y=w236) -> (x = y?=w255:bool)
    n80 = Greater?(x=w236, y=w258) -> (0:w254:bool)
    n81 = Select(t=w259, s=w255, f=w254) -> (s? t:f=w234:bool)
    "PWM Output 4" <- w234
    n82 = call "Plant System.vi"("Integrator ?"=w277, "Plant Input"=w236, "dt (s)"=w231, "process parameters"=w275) -> ("Plant Output"=w276:dbl)  [unwired: 11 in]
    n83 = Increment(x="Set Point 4") -> (x+1=w253:dbl)
    n84 = Decrement(x="Set Point 4") -> (x-1=w252:dbl)
    n85 = Select(t=w249, s=w234, f=w247) -> (s? t:f=w262:dbl)
    n86 = Select(t=w253, s=w234, f=w252) -> (s? t:f=w251:dbl)
    n87 = Not(x=w234) -> (.not. x?=w233:bool)
    n88 = call-poly <vilib>:"DAQmx Create Virtual Channel.vi"("lines"=tag "cDAQ1Mod1/port0/line3", "line grouping"=w240) -> ("task out"=w242:refnum<k21>, "error out"=w241:errorcluster)  [unwired: 12 in]
    n89 = call-poly <vilib>:"DAQmx Create Virtual Channel.vi"("lines"=tag "cDAQ1Mod2/port0/line3", "line grouping"=w222) -> ("task out"=w224:refnum<k21>, "error out"=w223:errorcluster)  [unwired: 12 in]
    n90 = Build Array(w229, "Set Point 4", w251) -> (w250:dbl[])
    n91 = Initialize Array("INLET 9 ON/OFF 2", 1 ("dimension size")) -> (w219:bool[])
    n92 = Initialize Array(w233, 1 ("dimension size")) -> (w237:bool[])
    n93 = local write "MV: 4"(w236) -> ()
    n94 = Add(x=w257, y=w260) -> (x+y=w261:dbl)
    n95 = Build Array(w250) -> (→"Real time Data 4":dbl[][])
    n96 = call-poly <vilib>:"DAQmx Write.vi"("task/channels in"=w242, "auto start"=TRUE, "data"=w237, "error in"=w241) -> ("task out"=w244:refnum<k21>, "error out"=w245:errorcluster)  [unwired: 9 in, 1 out]
    n97 = call-poly <vilib>:"DAQmx Write.vi"("task/channels in"=w224, "auto start"=TRUE, "data"=w219, "error in"=w223) -> ("task out"=w226:refnum<k21>, "error out"=w227:errorcluster)  [unwired: 9 in, 1 out]
    n98 = call <vilib>:"DAQmx Clear Task.vi"("task in"=w244, "error in"=w245) -> ("error out"=w239:errorcluster)  [unwired: 13 in]
    n99 = call <vilib>:"DAQmx Clear Task.vi"("task in"=w226, "error in"=w227) -> ("error out"=w221:errorcluster)  [unwired: 13 in]
    n100 = call <vilib>:"Simple Error Handler.vi"("error in (no error)"=w239) -> ()  [unwired: 4 in, 5 out]
    n101 = call <vilib>:"Simple Error Handler.vi"("error in (no error)"=w221) -> ()  [unwired: 4 in, 5 out]
  }
  n102 = while {
    shift-left: 0.0 ("Plant Output") -> [w374]
    shift-right: [w369] -> _
    tunnel: w73 -> [_]
    shift-right: [w355] -> _
    shift-left: 0.01 -> [w353]
    shift-right: [w327] -> _
    shift-left: TRUE -> [w352]
    shift-right: [w329] -> _
    shift-left: w70 -> [w351]
    shift-right: [w354] -> _
    shift-left: w70 -> [w350]
    tunnel: [w324] -> w69
    tunnel: w14 -> [w310]
    tunnel: [w309] -> w10
    stop <- "Stop 3" stop-if-true
    w315 = 1 items=["one channel for each line", "one channel for all lines"] ("line grouping")
    w324 = 0.05 ("Sampling Time dt (s)")
    w333 = 1 items=["one channel for each line", "one channel for all lines"] ("line grouping")
    w341 = 0.5 ("x")
    w368 = T7 {"static gain"=2.5, "lag (s)"=2.5, "deadtime (s)"=0.01, "load"=0.0, "deadband"=0.0, "sensor noise"=0.0, "initial PV"=30.0, "plant noise"=0.0}  # Process parameters
    w370 = FALSE  # Integrator ?
    # "C."
    # "Inlet 11"
    # "Exhaust 10"
    # "B."
    # "A."
    # "A.Output to PWM Logic \nB. Simulated Plant\nC. Draw Chart"
    # "Main PID Loop Control"
    n103 = Multiply(x=w324, y=1000.0) -> (x*y=w367:dbl)
    n104 = Not(x="Autotune 3") -> (.not. x?=w371:bool)
    n105 = feedback #5() -> (w376:bool)  [unwired: 1 in]
    n106 = feedback-in #5("Autotune 3") -> ()
    n107 = Wait Until Next ms Multiple(millisecond multiple=w367) -> ()  [unwired: 1 out]
    n108 = Exclusive Or(1:w376, 2:"Autotune 3") -> (0:w375:bool)
    n109 = feedback #6() -> (w373:dbl)  [unwired: 1 in]
    n110 = Multiply(x=w310, y=-1000.0) -> (x*y=w357:dynamicdata)
    n111 = call <vilib>:"Median PtByPt.vi"("sample length"="Median sample length 13", "x"=w357) -> ("median"=w356:dbl)  [unwired: 2 in, 1 out]
    n112 = Square(x=w356) -> (x^2=w364:dbl)
    n113 = Multiply(x=w356, y=-39.646) -> (x*y=w360:dbl)
    n114 = Multiply(x=w364, y=0.2324) -> (x*y=w361:dbl)
    n115 = Add(x=w360, y=w361) -> (x+y=w359:dbl)
    n116 = Add(x=1678.0, y=w359) -> (x+y=w322:dbl)
    n117 = case shown="False" "Autotune 3" {
      tunnel: w324 -> [w391 _]
      tunnel: [w380 w396] -> w329
      tunnel: w374 -> [_ w395]
      tunnel: "PID Gains 3" -> [w390 _]
      tunnel: "Reinitialize 3" -> [w387 _]
      tunnel: w375 -> [w389 w394]
      tunnel: w373 -> [_ w398]
      tunnel: w322 -> [w383 _]
      tunnel: "Set Point 3" -> [w382 _]
      frame False {
        # "This code is to have 'bumpless' transfer from autotuning"
        n118 = Not(x=w389) -> (.not. x?=w386:bool)
        n119 = And(x="Automatic 3", y=w386) -> (x .and. y?=w388:bool)
        n120 = call-poly <vilib>:"PID Advanced.vi"("setpoint"=w382, "auto? (T)"=w388, "manual control"="MV: 3", "process variable"=w383, "alpha"=10.0, "PID gains"=w390, "dt (s)"=w391, "reinitialize? (F)"=w387) -> ("output"=w380:dbl)  [unwired: 6 in, 1 out]
      }
      frame True {
        w401 = 10000 ("sample length")
        # "Buffering data for parameters estimation"
        n121 = call <vilib>:"Data Queue PtByPt.vi"("initial queue element"=w395, "initialize"=w394, "sample length"=w401, "input data point"=w395) -> ("Current Queue"=→"Control Output 3":dbl[])  [unwired: 3 in, 4 out]
        n122 = Select(t=0.0, s=w394, f="Excitation 3") -> (s? t:f=w399:dbl)
        n123 = Add(x=w398, y=w399) -> (x+y=w396:dbl)
        n124 = call <vilib>:"Data Queue PtByPt.vi"("initial queue element"=w396, "initialize"=w394, "sample length"=w401, "input data point"=w396) -> ("Current Queue"=→"Measurement 3":dbl[])  [unwired: 3 in, 4 out]
      }
    }
    n125 = feedback-in #6(w329, w371) -> ()
    n126 = Greater?(x=w322, y="M-10") -> (0:w309:bool)
    n127 = Add(x=w353, y=w341) -> (x+y=w342:dbl)
    n128 = Subtract(x=w353, y=w341) -> (x-y=w340:dbl)
    n129 = Equal?(x=w351, y=w329) -> (x = y?=w348:bool)
    n130 = Greater?(x=w329, y=w351) -> (0:w347:bool)
    n131 = Select(t=w352, s=w348, f=w347) -> (s? t:f=w327:bool)
    "PWM Output 3" <- w327
    n132 = call "Plant System.vi"("Integrator ?"=w370, "Plant Input"=w329, "dt (s)"=w324, "process parameters"=w368) -> ("Plant Output"=w369:dbl)  [unwired: 11 in]
    n133 = Increment(x="Set Point 3") -> (x+1=w346:dbl)
    n134 = Decrement(x="Set Point 3") -> (x-1=w345:dbl)
    n135 = Select(t=w342, s=w327, f=w340) -> (s? t:f=w355:dbl)
    n136 = Select(t=w346, s=w327, f=w345) -> (s? t:f=w344:dbl)
    n137 = Not(x=w327) -> (.not. x?=w326:bool)
    n138 = call-poly <vilib>:"DAQmx Create Virtual Channel.vi"("lines"=tag "cDAQ1Mod8/port0/line6", "line grouping"=w333) -> ("task out"=w335:refnum<k21>, "error out"=w334:errorcluster)  [unwired: 12 in]
    n139 = call-poly <vilib>:"DAQmx Create Virtual Channel.vi"("lines"=tag "cDAQ1Mod7/port0/line5", "line grouping"=w315) -> ("task out"=w317:refnum<k21>, "error out"=w316:errorcluster)  [unwired: 12 in]
    n140 = Build Array(w322, "Set Point 3", w344) -> (w343:dbl[])
    n141 = Initialize Array("INLET 10 ON/OFF", 1 ("dimension size")) -> (w312:bool[])
    n142 = Initialize Array(w326, 1 ("dimension size")) -> (w330:bool[])
    n143 = local write "MV: 3"(w329) -> ()
    n144 = Add(x=w350, y=w353) -> (x+y=w354:dbl)
    n145 = Build Array(w343) -> (→"Real time Data 3":dbl[][])
    n146 = call-poly <vilib>:"DAQmx Write.vi"("task/channels in"=w335, "auto start"=TRUE, "data"=w330, "error in"=w334) -> ("task out"=w337:refnum<k21>, "error out"=w338:errorcluster)  [unwired: 9 in, 1 out]
    n147 = call-poly <vilib>:"DAQmx Write.vi"("task/channels in"=w317, "auto start"=TRUE, "data"=w312, "error in"=w316) -> ("task out"=w319:refnum<k21>, "error out"=w320:errorcluster)  [unwired: 9 in, 1 out]
    n148 = call <vilib>:"DAQmx Clear Task.vi"("task in"=w337, "error in"=w338) -> ("error out"=w332:errorcluster)  [unwired: 13 in]
    n149 = call <vilib>:"DAQmx Clear Task.vi"("task in"=w319, "error in"=w320) -> ("error out"=w314:errorcluster)  [unwired: 13 in]
    n150 = call <vilib>:"Simple Error Handler.vi"("error in (no error)"=w332) -> ()  [unwired: 4 in, 5 out]
    n151 = call <vilib>:"Simple Error Handler.vi"("error in (no error)"=w314) -> ()  [unwired: 4 in, 5 out]
  }
  n152 = while {
    shift-left: 0.0 ("Plant Output") -> [w467]
    shift-right: [w462] -> _
    tunnel: w61 -> [_]
    shift-right: [w448] -> _
    shift-left: 0.01 -> [w446]
    shift-right: [w420] -> _
    shift-left: TRUE -> [w445]
    shift-right: [w422] -> _
    shift-left: w58 -> [w444]
    shift-right: [w447] -> _
    shift-left: w58 -> [w443]
    tunnel: [w417] -> w57
    tunnel: w14 -> [w403]
    tunnel: [w402] -> w8
    stop <- "Stop 5" stop-if-true
    w408 = 1 items=["one channel for each line", "one channel for all lines"] ("line grouping")
    w417 = 0.05 ("Sampling Time dt (s)")
    w426 = 1 items=["one channel for each line", "one channel for all lines"] ("line grouping")
    w434 = 0.5 ("x")
    w461 = T7 {"static gain"=2.5, "lag (s)"=2.5, "deadtime (s)"=0.01, "load"=0.0, "deadband"=0.0, "sensor noise"=0.0, "initial PV"=30.0, "plant noise"=0.0}  # Process parameters
    w463 = FALSE  # Integrator ?
    # "C."
    # "Inlet 11"
    # "Exhaust 8"
    # "B."
    # "A."
    # "A.Output to PWM Logic \nB. Simulated Plant\nC. Draw Chart"
    # "Main PID Loop Control"
    n153 = Multiply(x=w417, y=1000.0) -> (x*y=w460:dbl)
    n154 = Not(x="Autotune 5") -> (.not. x?=w464:bool)
    n155 = feedback #7() -> (w469:bool)  [unwired: 1 in]
    n156 = feedback-in #7("Autotune 5") -> ()
    n157 = Wait Until Next ms Multiple(millisecond multiple=w460) -> ()  [unwired: 1 out]
    n158 = Exclusive Or(1:w469, 2:"Autotune 5") -> (0:w468:bool)
    n159 = feedback #8() -> (w466:dbl)  [unwired: 1 in]
    n160 = Multiply(x=w403, y=-1000.0) -> (x*y=w450:dynamicdata)
    n161 = call <vilib>:"Median PtByPt.vi"("sample length"="Median sample length 14", "x"=w450) -> ("median"=w449:dbl)  [unwired: 2 in, 1 out]
    n162 = Square(x=w449) -> (x^2=w457:dbl)
    n163 = Multiply(x=w449, y=-39.646) -> (x*y=w453:dbl)
    n164 = Multiply(x=w457, y=0.2324) -> (x*y=w454:dbl)
    n165 = Add(x=w453, y=w454) -> (x+y=w452:dbl)
    n166 = Add(x=1678.0, y=w452) -> (x+y=w415:dbl)
    n167 = case shown="False" "Autotune 5" {
      tunnel: w417 -> [w484 _]
      tunnel: [w473 w489] -> w422
      tunnel: w467 -> [_ w488]
      tunnel: "PID Gains 5" -> [w483 _]
      tunnel: "Reinitialize 5" -> [w480 _]
      tunnel: w468 -> [w482 w487]
      tunnel: w466 -> [_ w491]
      tunnel: w415 -> [w476 _]
      tunnel: "Set Point 5" -> [w475 _]
      frame False {
        # "This code is to have 'bumpless' transfer from autotuning"
        n168 = Not(x=w482) -> (.not. x?=w479:bool)
        n169 = And(x="Automatic 5", y=w479) -> (x .and. y?=w481:bool)
        n170 = call-poly <vilib>:"PID Advanced.vi"("setpoint"=w475, "auto? (T)"=w481, "manual control"="MV: 5", "process variable"=w476, "alpha"=10.0, "PID gains"=w483, "dt (s)"=w484, "reinitialize? (F)"=w480) -> ("output"=w473:dbl)  [unwired: 6 in, 1 out]
      }
      frame True {
        w494 = 10000 ("sample length")
        # "Buffering data for parameters estimation"
        n171 = call <vilib>:"Data Queue PtByPt.vi"("initial queue element"=w488, "initialize"=w487, "sample length"=w494, "input data point"=w488) -> ("Current Queue"=→"Control Output 5":dbl[])  [unwired: 3 in, 4 out]
        n172 = Select(t=0.0, s=w487, f="Excitation 5") -> (s? t:f=w492:dbl)
        n173 = Add(x=w491, y=w492) -> (x+y=w489:dbl)
        n174 = call <vilib>:"Data Queue PtByPt.vi"("initial queue element"=w489, "initialize"=w487, "sample length"=w494, "input data point"=w489) -> ("Current Queue"=→"Measurement 5":dbl[])  [unwired: 3 in, 4 out]
      }
    }
    n175 = feedback-in #8(w422, w464) -> ()
    n176 = Greater?(x=w415, y="M-8") -> (0:w402:bool)
    n177 = Add(x=w446, y=w434) -> (x+y=w435:dbl)
    n178 = Subtract(x=w446, y=w434) -> (x-y=w433:dbl)
    n179 = Equal?(x=w444, y=w422) -> (x = y?=w441:bool)
    n180 = Greater?(x=w422, y=w444) -> (0:w440:bool)
    n181 = Select(t=w445, s=w441, f=w440) -> (s? t:f=w420:bool)
    "PWM Output 5" <- w420
    n182 = call "Plant System.vi"("Integrator ?"=w463, "Plant Input"=w422, "dt (s)"=w417, "process parameters"=w461) -> ("Plant Output"=w462:dbl)  [unwired: 11 in]
    n183 = Increment(x="Set Point 5") -> (x+1=w439:dbl)
    n184 = Decrement(x="Set Point 5") -> (x-1=w438:dbl)
    n185 = Select(t=w435, s=w420, f=w433) -> (s? t:f=w448:dbl)
    n186 = Select(t=w439, s=w420, f=w438) -> (s? t:f=w437:dbl)
    n187 = Not(x=w420) -> (.not. x?=w419:bool)
    n188 = call-poly <vilib>:"DAQmx Create Virtual Channel.vi"("lines"=tag "cDAQ1Mod8/port0/line3", "line grouping"=w426) -> ("task out"=w428:refnum<k21>, "error out"=w427:errorcluster)  [unwired: 12 in]
    n189 = call-poly <vilib>:"DAQmx Create Virtual Channel.vi"("lines"=tag "cDAQ1Mod7/port0/line2", "line grouping"=w408) -> ("task out"=w410:refnum<k21>, "error out"=w409:errorcluster)  [unwired: 12 in]
    n190 = Build Array(w415, "Set Point 5", w437) -> (w436:dbl[])
    n191 = Initialize Array("INLET 8 ON/OFF 2", 1 ("dimension size")) -> (w405:bool[])
    n192 = Initialize Array(w419, 1 ("dimension size")) -> (w423:bool[])
    n193 = local write "MV: 5"(w422) -> ()
    n194 = Add(x=w443, y=w446) -> (x+y=w447:dbl)
    n195 = Build Array(w436) -> (→"Real time Data 5":dbl[][])
    n196 = call-poly <vilib>:"DAQmx Write.vi"("task/channels in"=w428, "auto start"=TRUE, "data"=w423, "error in"=w427) -> ("task out"=w430:refnum<k21>, "error out"=w431:errorcluster)  [unwired: 9 in, 1 out]
    n197 = call-poly <vilib>:"DAQmx Write.vi"("task/channels in"=w410, "auto start"=TRUE, "data"=w405, "error in"=w409) -> ("task out"=w412:refnum<k21>, "error out"=w413:errorcluster)  [unwired: 9 in, 1 out]
    n198 = call <vilib>:"DAQmx Clear Task.vi"("task in"=w430, "error in"=w431) -> ("error out"=w425:errorcluster)  [unwired: 13 in]
    n199 = call <vilib>:"DAQmx Clear Task.vi"("task in"=w412, "error in"=w413) -> ("error out"=w407:errorcluster)  [unwired: 13 in]
    n200 = call <vilib>:"Simple Error Handler.vi"("error in (no error)"=w425) -> ()  [unwired: 4 in, 5 out]
    n201 = call <vilib>:"Simple Error Handler.vi"("error in (no error)"=w407) -> ()  [unwired: 4 in, 5 out]
  }
  n202 = while {
    shift-left: 0.0 ("Plant Output") -> [w560]
    shift-right: [w555] -> _
    tunnel: w79 -> [_]
    shift-right: [w541] -> _
    shift-left: 0.01 -> [w539]
    shift-right: [w513] -> _
    shift-left: TRUE -> [w538]
    shift-right: [w515] -> _
    shift-left: w76 -> [w537]
    shift-right: [w540] -> _
    shift-left: w76 -> [w536]
    tunnel: [w510] -> w75
    tunnel: w14 -> [w496]
    tunnel: [w495] -> w11
    stop <- "Stop 2" stop-if-true
    w501 = 1 items=["one channel for each line", "one channel for all lines"] ("line grouping")
    w510 = 0.05 ("Sampling Time dt (s)")
    w519 = 1 items=["one channel for each line", "one channel for all lines"] ("line grouping")
    w527 = 0.5 ("x")
    w554 = T7 {"static gain"=2.5, "lag (s)"=2.5, "deadtime (s)"=0.01, "load"=0.0, "deadband"=0.0, "sensor noise"=0.0, "initial PV"=30.0, "plant noise"=0.0}  # Process parameters
    w556 = FALSE  # Integrator ?
    # "C."
    # "Inlet 11"
    # "Exhaust 12"
    # "B."
    # "A."
    # "A.Output to PWM Logic \nB. Simulated Plant\nC. Draw Chart"
    # "Main PID Loop Control"
    n203 = Multiply(x=w510, y=1000.0) -> (x*y=w553:dbl)
    n204 = Not(x="Autotune 2") -> (.not. x?=w557:bool)
    n205 = feedback #9() -> (w562:bool)  [unwired: 1 in]
    n206 = feedback-in #9("Autotune 2") -> ()
    n207 = Wait Until Next ms Multiple(millisecond multiple=w553) -> ()  [unwired: 1 out]
    n208 = Exclusive Or(1:w562, 2:"Autotune 2") -> (0:w561:bool)
    n209 = feedback #10() -> (w559:dbl)  [unwired: 1 in]
    n210 = Multiply(x=w496, y=-1000.0) -> (x*y=w543:dynamicdata)
    n211 = call <vilib>:"Median PtByPt.vi"("sample length"="Median sample length 12", "x"=w543) -> ("median"=w542:dbl)  [unwired: 2 in, 1 out]
    n212 = Square(x=w542) -> (x^2=w550:dbl)
    n213 = Multiply(x=w542, y=-39.646) -> (x*y=w546:dbl)
    n214 = Multiply(x=w550, y=0.2324) -> (x*y=w547:dbl)
    n215 = Add(x=w546, y=w547) -> (x+y=w545:dbl)
    n216 = Add(x=1678.0, y=w545) -> (x+y=w508:dbl)
    n217 = case shown="False" "Autotune 2" {
      tunnel: w510 -> [w577 _]
      tunnel: [w566 w582] -> w515
      tunnel: w560 -> [_ w581]
      tunnel: "PID Gains 2" -> [w576 _]
      tunnel: "Reinitialize 2" -> [w573 _]
      tunnel: w561 -> [w575 w580]
      tunnel: w559 -> [_ w584]
      tunnel: w508 -> [w569 _]
      tunnel: "Set Point 2" -> [w568 _]
      frame False {
        # "This code is to have 'bumpless' transfer from autotuning"
        n218 = Not(x=w575) -> (.not. x?=w572:bool)
        n219 = And(x="Automatic 2", y=w572) -> (x .and. y?=w574:bool)
        n220 = call-poly <vilib>:"PID Advanced.vi"("setpoint"=w568, "auto? (T)"=w574, "manual control"="MV: 2", "process variable"=w569, "alpha"=10.0, "PID gains"=w576, "dt (s)"=w577, "reinitialize? (F)"=w573) -> ("output"=w566:dbl)  [unwired: 6 in, 1 out]
      }
      frame True {
        w587 = 10000 ("sample length")
        # "Buffering data for parameters estimation"
        n221 = call <vilib>:"Data Queue PtByPt.vi"("initial queue element"=w581, "initialize"=w580, "sample length"=w587, "input data point"=w581) -> ("Current Queue"=→"Control Output 2":dbl[])  [unwired: 3 in, 4 out]
        n222 = Select(t=0.0, s=w580, f="Excitation 2") -> (s? t:f=w585:dbl)
        n223 = Add(x=w584, y=w585) -> (x+y=w582:dbl)
        n224 = call <vilib>:"Data Queue PtByPt.vi"("initial queue element"=w582, "initialize"=w580, "sample length"=w587, "input data point"=w582) -> ("Current Queue"=→"Measurement 2":dbl[])  [unwired: 3 in, 4 out]
      }
    }
    n225 = feedback-in #10(w515, w557) -> ()
    n226 = Greater?(x=w508, y="M-12") -> (0:w495:bool)
    n227 = Add(x=w539, y=w527) -> (x+y=w528:dbl)
    n228 = Subtract(x=w539, y=w527) -> (x-y=w526:dbl)
    n229 = Equal?(x=w537, y=w515) -> (x = y?=w534:bool)
    n230 = Greater?(x=w515, y=w537) -> (0:w533:bool)
    n231 = Select(t=w538, s=w534, f=w533) -> (s? t:f=w513:bool)
    "PWM Output 2" <- w513
    n232 = call "Plant System.vi"("Integrator ?"=w556, "Plant Input"=w515, "dt (s)"=w510, "process parameters"=w554) -> ("Plant Output"=w555:dbl)  [unwired: 11 in]
    n233 = Increment(x="Set Point 2") -> (x+1=w532:dbl)
    n234 = Decrement(x="Set Point 2") -> (x-1=w531:dbl)
    n235 = Select(t=w528, s=w513, f=w526) -> (s? t:f=w541:dbl)
    n236 = Select(t=w532, s=w513, f=w531) -> (s? t:f=w530:dbl)
    n237 = Not(x=w513) -> (.not. x?=w512:bool)
    n238 = call-poly <vilib>:"DAQmx Create Virtual Channel.vi"("lines"=tag "cDAQ1Mod8/port0/line2", "line grouping"=w519) -> ("task out"=w521:refnum<k21>, "error out"=w520:errorcluster)  [unwired: 12 in]
    n239 = call-poly <vilib>:"DAQmx Create Virtual Channel.vi"("lines"=tag "cDAQ1Mod7/port0/line1", "line grouping"=w501) -> ("task out"=w503:refnum<k21>, "error out"=w502:errorcluster)  [unwired: 12 in]
    n240 = Build Array(w508, "Set Point 2", w530) -> (w529:dbl[])
    n241 = Initialize Array("INLET 12 ON/OFF", 1 ("dimension size")) -> (w498:bool[])
    n242 = Initialize Array(w512, 1 ("dimension size")) -> (w516:bool[])
    n243 = local write "MV: 2"(w515) -> ()
    n244 = Add(x=w536, y=w539) -> (x+y=w540:dbl)
    n245 = Build Array(w529) -> (→"Real time Data 2":dbl[][])
    n246 = call-poly <vilib>:"DAQmx Write.vi"("task/channels in"=w521, "auto start"=TRUE, "data"=w516, "error in"=w520) -> ("task out"=w523:refnum<k21>, "error out"=w524:errorcluster)  [unwired: 9 in, 1 out]
    n247 = call-poly <vilib>:"DAQmx Write.vi"("task/channels in"=w503, "auto start"=TRUE, "data"=w498, "error in"=w502) -> ("task out"=w505:refnum<k21>, "error out"=w506:errorcluster)  [unwired: 9 in, 1 out]
    n248 = call <vilib>:"DAQmx Clear Task.vi"("task in"=w523, "error in"=w524) -> ("error out"=w518:errorcluster)  [unwired: 13 in]
    n249 = call <vilib>:"DAQmx Clear Task.vi"("task in"=w505, "error in"=w506) -> ("error out"=w500:errorcluster)  [unwired: 13 in]
    n250 = call <vilib>:"Simple Error Handler.vi"("error in (no error)"=w518) -> ()  [unwired: 4 in, 5 out]
    n251 = call <vilib>:"Simple Error Handler.vi"("error in (no error)"=w500) -> ()  [unwired: 4 in, 5 out]
  }
  n252 = while {
    shift-left: 0.0 ("Plant Output") -> [w653]
    shift-right: [w648] -> _
    tunnel: w121 -> [_]
    shift-right: [w634] -> _
    shift-left: 0.01 -> [w632]
    shift-right: [w606] -> _
    shift-left: TRUE -> [w631]
    shift-right: [w608] -> _
    shift-left: w118 -> [w630]
    shift-right: [w633] -> _
    shift-left: w118 -> [w629]
    tunnel: [w603] -> w117
    tunnel: [w600] -> w13
    tunnel: w14 -> [w588]
    stop <- "Stop" stop-if-true
    w593 = 1 items=["one channel for each line", "one channel for all lines"] ("line grouping")
    w603 = 0.05 ("Sampling Time dt (s)")
    w612 = 1 items=["one channel for each line", "one channel for all lines"] ("line grouping")
    w620 = 0.5 ("x")
    w647 = T7 {"static gain"=2.5, "lag (s)"=2.5, "deadtime (s)"=0.01, "load"=0.0, "deadband"=0.0, "sensor noise"=0.0, "initial PV"=30.0, "plant noise"=0.0}  # Process parameters
    w649 = FALSE  # Integrator ?
    # "C."
    # "Inlet 11"
    # "Exhaust 11"
    # "B."
    # "A."
    # "A.Output to PWM Logic \nB. Simulated Plant\nC. Draw Chart"
    # "Main PID Loop Control"
    n253 = Multiply(x=w603, y=1000.0) -> (x*y=w646:dbl)
    n254 = Not(x="Autotune") -> (.not. x?=w650:bool)
    n255 = feedback #11() -> (w655:bool)  [unwired: 1 in]
    n256 = feedback-in #11("Autotune") -> ()
    n257 = Wait Until Next ms Multiple(millisecond multiple=w646) -> ()  [unwired: 1 out]
    n258 = Exclusive Or(1:w655, 2:"Autotune") -> (0:w654:bool)
    n259 = feedback #12() -> (w652:dbl)  [unwired: 1 in]
    n260 = Multiply(x=w588, y=-1000.0) -> (x*y=w636:dynamicdata)
    n261 = call <vilib>:"Median PtByPt.vi"("sample length"="Median sample length", "x"=w636) -> ("median"=w635:dbl)  [unwired: 2 in, 1 out]
    n262 = Square(x=w635) -> (x^2=w643:dbl)
    n263 = Multiply(x=w635, y=-39.646) -> (x*y=w639:dbl)
    n264 = Multiply(x=w643, y=0.2324) -> (x*y=w640:dbl)
    n265 = Add(x=w639, y=w640) -> (x+y=w638:dbl)
    n266 = Add(x=1678.0, y=w638) -> (x+y=w601:dbl)
    n267 = case shown="False" "Autotune" {
      tunnel: w603 -> [w670 _]
      tunnel: [w659 w675] -> w608
      tunnel: w653 -> [_ w674]
      tunnel: "PID Gains" -> [w669 _]
      tunnel: "Reinitialize" -> [w666 _]
      tunnel: w654 -> [w668 w673]
      tunnel: w652 -> [_ w677]
      tunnel: w601 -> [w662 _]
      tunnel: "Set Point" -> [w661 _]
      frame False {
        # "This code is to have 'bumpless' transfer from autotuning"
        n268 = Not(x=w668) -> (.not. x?=w665:bool)
        n269 = And(x="Automatic", y=w665) -> (x .and. y?=w667:bool)
        n270 = call-poly <vilib>:"PID Advanced.vi"("setpoint"=w661, "auto? (T)"=w667, "manual control"="MV:", "process variable"=w662, "alpha"=10.0, "PID gains"=w669, "dt (s)"=w670, "reinitialize? (F)"=w666) -> ("output"=w659:dbl)  [unwired: 6 in, 1 out]
      }
      frame True {
        w680 = 10000 ("sample length")
        # "Buffering data for parameters estimation"
        n271 = call <vilib>:"Data Queue PtByPt.vi"("initial queue element"=w674, "initialize"=w673, "sample length"=w680, "input data point"=w674) -> ("Current Queue"=→"Control Output":dbl[])  [unwired: 3 in, 4 out]
        n272 = Select(t=0.0, s=w673, f="Excitation") -> (s? t:f=w678:dbl)
        n273 = Add(x=w677, y=w678) -> (x+y=w675:dbl)
        n274 = call <vilib>:"Data Queue PtByPt.vi"("initial queue element"=w675, "initialize"=w673, "sample length"=w680, "input data point"=w675) -> ("Current Queue"=→"Measurement":dbl[])  [unwired: 3 in, 4 out]
      }
    }
    n275 = feedback-in #12(w608, w650) -> ()
    n276 = Greater?(x=w601, y="M-11") -> (0:w600:bool)
    n277 = Add(x=w632, y=w620) -> (x+y=w621:dbl)
    n278 = Subtract(x=w632, y=w620) -> (x-y=w619:dbl)
    n279 = Equal?(x=w630, y=w608) -> (x = y?=w627:bool)
    n280 = Greater?(x=w608, y=w630) -> (0:w626:bool)
    n281 = Select(t=w631, s=w627, f=w626) -> (s? t:f=w606:bool)
    "PWM Output" <- w606
    n282 = call "Plant System.vi"("Integrator ?"=w649, "Plant Input"=w608, "dt (s)"=w603, "process parameters"=w647) -> ("Plant Output"=w648:dbl)  [unwired: 11 in]
    n283 = Increment(x="Set Point") -> (x+1=w625:dbl)
    n284 = Decrement(x="Set Point") -> (x-1=w624:dbl)
    n285 = Select(t=w621, s=w606, f=w619) -> (s? t:f=w634:dbl)
    n286 = Select(t=w625, s=w606, f=w624) -> (s? t:f=w623:dbl)
    n287 = Not(x=w606) -> (.not. x?=w605:bool)
    n288 = call-poly <vilib>:"DAQmx Create Virtual Channel.vi"("lines"=tag "cDAQ1Mod1/port0/line2", "line grouping"=w612) -> ("task out"=w614:refnum<k21>, "error out"=w613:errorcluster)  [unwired: 12 in]
    n289 = call-poly <vilib>:"DAQmx Create Virtual Channel.vi"("lines"=tag "cDAQ1Mod2/port0/line2", "line grouping"=w593) -> ("task out"=w595:refnum<k21>, "error out"=w594:errorcluster)  [unwired: 12 in]
    n290 = Build Array(w601, "Set Point", w623) -> (w622:dbl[])
    n291 = Initialize Array("INLET", 1 ("dimension size")) -> (w590:bool[])
    n292 = Initialize Array(w605, 1 ("dimension size")) -> (w609:bool[])
    n293 = local write "MV:"(w608) -> ()
    n294 = Add(x=w629, y=w632) -> (x+y=w633:dbl)
    n295 = Build Array(w622) -> (→"Real time Data":dbl[][])
    n296 = call-poly <vilib>:"DAQmx Write.vi"("task/channels in"=w614, "auto start"=TRUE, "data"=w609, "error in"=w613) -> ("task out"=w616:refnum<k21>, "error out"=w617:errorcluster)  [unwired: 9 in, 1 out]
    n297 = call-poly <vilib>:"DAQmx Write.vi"("task/channels in"=w595, "auto start"=TRUE, "data"=w590, "error in"=w594) -> ("task out"=w597:refnum<k21>, "error out"=w598:errorcluster)  [unwired: 9 in, 1 out]
    n298 = call <vilib>:"DAQmx Clear Task.vi"("task in"=w616, "error in"=w617) -> ("error out"=w611:errorcluster)  [unwired: 13 in]
    n299 = call <vilib>:"DAQmx Clear Task.vi"("task in"=w597, "error in"=w598) -> ("error out"=w592:errorcluster)  [unwired: 13 in]
    n300 = call <vilib>:"Simple Error Handler.vi"("error in (no error)"=w611) -> ()  [unwired: 4 in, 5 out]
    n301 = call <vilib>:"Simple Error Handler.vi"("error in (no error)"=w592) -> ()  [unwired: 4 in, 5 out]
  }
  n302 = local write "Stop 6"(w55) -> ()
  n303 = local write "Stop 4"(w67) -> ()
  n304 = local write "Stop 3"(w73) -> ()
  n305 = local write "Stop 5"(w61) -> ()
  n306 = local write "Stop 2"(w79) -> ()
  n307 = local write "Stop"(w121) -> ()
  n308 = call-poly "VISA Configure Serial Port"("VISA resource name"="COM Port-Sensor 1") -> ("VISA resource name out"=w112:refnum<visa-resource-name>, "error out"=w111:errorcluster)  [unwired: 9 in, 4 out]
  n309 = call-poly "VISA Configure Serial Port"("VISA resource name"="COM Port-Sensor 2") -> ("VISA resource name out"=w107:refnum<visa-resource-name>, "error out"=w106:errorcluster)  [unwired: 9 in, 4 out]
  n310 = while {
    tunnel: w55 -> [_]
    tunnel: w51 -> [w684]
    stop <- w694 stop-if-true
    # "If dT and deadtime have similar values, the identification could evaluate deadtime as zero and this generates proportional gain equal to Inf. This code avoid gain changes in this situations."
    # "Autotuning Loop"
    n311 = local read "Control Output 6"() -> (w696:dbl[])
    n312 = local read "Measurement 6"() -> (w695:dbl[])
    n313 = case shown="\"Chien-Hrones-Reswick\"" "Control 6" {
      tunnel: w696 -> [w705 w713 w722 w731]
      tunnel: w695 -> [w704 w712 w721 w730]
      tunnel: [w703 w711 w720 w729] -> w683
      tunnel: [w702 w710 w719 w728] -> w682
      tunnel: w684 -> [w701 w709 w718 w727]
      tunnel: [w700 w708 w717 w726] -> w681
      tunnel: [w699 w707 w716 w725] -> w686
      tunnel: "Type of controller 6" -> [w698 w706 w715 w724]
      frame "Ziegler-Nichols", Default {
        n314 = call-poly <vilib>:"PID Autotuning Design.vi"("Ziegler-Nichols Speed"="Ziegler-Nichols speed 6", "Type of Controller"=w698, "dt (s)"=w701, "Response signal"=w704, "Stimulus signal"=w705) -> ("PID gains"=w699:T2, "response operating point"=w702:dbl, "stimulus operating point"=w703:dbl, "Plant Parameters"=w700:T4)  [unwired: 3 in]
      }
      frame "Cohen-Coon" {
        n315 = call-poly <vilib>:"PID Autotuning Design.vi"("Type of Controller"=w706, "dt (s)"=w709, "Response signal"=w712, "Stimulus signal"=w713) -> ("PID gains"=w707:T2, "response offset"=w710:dbl, "stimulus offset"=w711:dbl, "Plant Parameters"=w708:T4)  [unwired: 4 in]
      }
      frame "Chien-Hrones-Reswick" {
        n316 = call-poly <vilib>:"PID Autotuning Design.vi"("Tuning specifications"="Tuning specifications 6", "Type of Controller"=w715, "dt (s)"=w718, "Response signal"=w721, "Stimulus signal"=w722) -> ("PID gains"=w716:T2, "response offset"=w719:dbl, "stimulus offset"=w720:dbl, "Plant Parameters"=w717:T4)  [unwired: 3 in]
      }
      frame "Internal Model Control" {
        n317 = call-poly <vilib>:"PID Autotuning Design.vi"("Desired Time Constant (tau_c)"="Multiplicative factor 6", "Type of Controller"=w724, "dt (s)"=w727, "Response signal"=w730, "Stimulus signal"=w731) -> ("PID gains"=w725:T2, "response offset"=w728:dbl, "stimulus offset"=w729:dbl, "Plant Parameters"=w726:T4)  [unwired: 3 in]
      }
    }
    "Stimulus operating point 6" <- w683
    "Response operating point 6" <- w682
    "Identified Plant Parameters 6" <- w681
    n318 = Unbundle(w686) -> ("proportional gain (Kc)"=w689:dbl)  [unwired: 2 out]
    n319 = Equal?(x=w689, y=inf) -> (x = y?=w688:bool)
    n320 = feedback #13() -> (w687:T2)  [unwired: 1 in]
    n321 = Select(t=w687, s=w688, f=w686) -> (s? t:f=w685:T2)
    "Tuned PID gains 6" <- w685
    n322 = feedback-in #13(w685) -> ()
    n323 = case shown="True" "Accept gain 6" {
      tunnel: w685 -> [_ w732]
      frame False {
      }
      frame True {
        n324 = local write "PID Gains 6"(w732) -> ()
      }
    }
    n325 = local read "Stop 6"() -> (w694:bool)
  }
  n326 = while {
    tunnel: w67 -> [_]
    tunnel: w63 -> [w736]
    stop <- w746 stop-if-true
    # "If dT and deadtime have similar values, the identification could evaluate deadtime as zero and this generates proportional gain equal to Inf. This code avoid gain changes in this situations."
    # "Autotuning Loop"
    n327 = local read "Control Output 4"() -> (w748:dbl[])
    n328 = local read "Measurement 4"() -> (w747:dbl[])
    n329 = case shown="\"Chien-Hrones-Reswick\"" "Control 4" {
      tunnel: w748 -> [w757 w765 w774 w783]
      tunnel: w747 -> [w756 w764 w773 w782]
      tunnel: [w755 w763 w772 w781] -> w735
      tunnel: [w754 w762 w771 w780] -> w734
      tunnel: w736 -> [w753 w761 w770 w779]
      tunnel: [w752 w760 w769 w778] -> w733
      tunnel: [w751 w759 w768 w777] -> w738
      tunnel: "Type of controller 4" -> [w750 w758 w767 w776]
      frame "Ziegler-Nichols", Default {
        n330 = call-poly <vilib>:"PID Autotuning Design.vi"("Ziegler-Nichols Speed"="Ziegler-Nichols speed 4", "Type of Controller"=w750, "dt (s)"=w753, "Response signal"=w756, "Stimulus signal"=w757) -> ("PID gains"=w751:T2, "response operating point"=w754:dbl, "stimulus operating point"=w755:dbl, "Plant Parameters"=w752:T4)  [unwired: 3 in]
      }
      frame "Cohen-Coon" {
        n331 = call-poly <vilib>:"PID Autotuning Design.vi"("Type of Controller"=w758, "dt (s)"=w761, "Response signal"=w764, "Stimulus signal"=w765) -> ("PID gains"=w759:T2, "response offset"=w762:dbl, "stimulus offset"=w763:dbl, "Plant Parameters"=w760:T4)  [unwired: 4 in]
      }
      frame "Chien-Hrones-Reswick" {
        n332 = call-poly <vilib>:"PID Autotuning Design.vi"("Tuning specifications"="Tuning specifications 4", "Type of Controller"=w767, "dt (s)"=w770, "Response signal"=w773, "Stimulus signal"=w774) -> ("PID gains"=w768:T2, "response offset"=w771:dbl, "stimulus offset"=w772:dbl, "Plant Parameters"=w769:T4)  [unwired: 3 in]
      }
      frame "Internal Model Control" {
        n333 = call-poly <vilib>:"PID Autotuning Design.vi"("Desired Time Constant (tau_c)"="Multiplicative factor 4", "Type of Controller"=w776, "dt (s)"=w779, "Response signal"=w782, "Stimulus signal"=w783) -> ("PID gains"=w777:T2, "response offset"=w780:dbl, "stimulus offset"=w781:dbl, "Plant Parameters"=w778:T4)  [unwired: 3 in]
      }
    }
    "Stimulus operating point 4" <- w735
    "Response operating point 4" <- w734
    "Identified Plant Parameters 4" <- w733
    n334 = Unbundle(w738) -> ("proportional gain (Kc)"=w741:dbl)  [unwired: 2 out]
    n335 = Equal?(x=w741, y=inf) -> (x = y?=w740:bool)
    n336 = feedback #14() -> (w739:T2)  [unwired: 1 in]
    n337 = Select(t=w739, s=w740, f=w738) -> (s? t:f=w737:T2)
    "Tuned PID gains 4" <- w737
    n338 = feedback-in #14(w737) -> ()
    n339 = case shown="True" "Accept gain 4" {
      tunnel: w737 -> [_ w784]
      frame False {
      }
      frame True {
        n340 = local write "PID Gains 4"(w784) -> ()
      }
    }
    n341 = local read "Stop 4"() -> (w746:bool)
  }
  n342 = while {
    tunnel: w73 -> [_]
    tunnel: w69 -> [w788]
    stop <- w798 stop-if-true
    # "If dT and deadtime have similar values, the identification could evaluate deadtime as zero and this generates proportional gain equal to Inf. This code avoid gain changes in this situations."
    # "Autotuning Loop"
    n343 = local read "Control Output 3"() -> (w800:dbl[])
    n344 = local read "Measurement 3"() -> (w799:dbl[])
    n345 = case shown="\"Chien-Hrones-Reswick\"" "Control 3" {
      tunnel: w800 -> [w809 w817 w826 w835]
      tunnel: w799 -> [w808 w816 w825 w834]
      tunnel: [w807 w815 w824 w833] -> w787
      tunnel: [w806 w814 w823 w832] -> w786
      tunnel: w788 -> [w805 w813 w822 w831]
      tunnel: [w804 w812 w821 w830] -> w785
      tunnel: [w803 w811 w820 w829] -> w790
      tunnel: "Type of controller 3" -> [w802 w810 w819 w828]
      frame "Ziegler-Nichols", Default {
        n346 = call-poly <vilib>:"PID Autotuning Design.vi"("Ziegler-Nichols Speed"="Ziegler-Nichols speed 3", "Type of Controller"=w802, "dt (s)"=w805, "Response signal"=w808, "Stimulus signal"=w809) -> ("PID gains"=w803:T2, "response operating point"=w806:dbl, "stimulus operating point"=w807:dbl, "Plant Parameters"=w804:T4)  [unwired: 3 in]
      }
      frame "Cohen-Coon" {
        n347 = call-poly <vilib>:"PID Autotuning Design.vi"("Type of Controller"=w810, "dt (s)"=w813, "Response signal"=w816, "Stimulus signal"=w817) -> ("PID gains"=w811:T2, "response offset"=w814:dbl, "stimulus offset"=w815:dbl, "Plant Parameters"=w812:T4)  [unwired: 4 in]
      }
      frame "Chien-Hrones-Reswick" {
        n348 = call-poly <vilib>:"PID Autotuning Design.vi"("Tuning specifications"="Tuning specifications 3", "Type of Controller"=w819, "dt (s)"=w822, "Response signal"=w825, "Stimulus signal"=w826) -> ("PID gains"=w820:T2, "response offset"=w823:dbl, "stimulus offset"=w824:dbl, "Plant Parameters"=w821:T4)  [unwired: 3 in]
      }
      frame "Internal Model Control" {
        n349 = call-poly <vilib>:"PID Autotuning Design.vi"("Desired Time Constant (tau_c)"="Multiplicative factor 3", "Type of Controller"=w828, "dt (s)"=w831, "Response signal"=w834, "Stimulus signal"=w835) -> ("PID gains"=w829:T2, "response offset"=w832:dbl, "stimulus offset"=w833:dbl, "Plant Parameters"=w830:T4)  [unwired: 3 in]
      }
    }
    "Stimulus operating point 3" <- w787
    "Response operating point 3" <- w786
    "Identified Plant Parameters 3" <- w785
    n350 = Unbundle(w790) -> ("proportional gain (Kc)"=w793:dbl)  [unwired: 2 out]
    n351 = Equal?(x=w793, y=inf) -> (x = y?=w792:bool)
    n352 = feedback #15() -> (w791:T2)  [unwired: 1 in]
    n353 = Select(t=w791, s=w792, f=w790) -> (s? t:f=w789:T2)
    "Tuned PID gains 3" <- w789
    n354 = feedback-in #15(w789) -> ()
    n355 = case shown="True" "Accept gain 3" {
      tunnel: w789 -> [_ w836]
      frame False {
      }
      frame True {
        n356 = local write "PID Gains 3"(w836) -> ()
      }
    }
    n357 = local read "Stop 3"() -> (w798:bool)
  }
  n358 = while {
    tunnel: w61 -> [_]
    tunnel: w57 -> [w840]
    stop <- w850 stop-if-true
    # "If dT and deadtime have similar values, the identification could evaluate deadtime as zero and this generates proportional gain equal to Inf. This code avoid gain changes in this situations."
    # "Autotuning Loop"
    n359 = local read "Control Output 5"() -> (w852:dbl[])
    n360 = local read "Measurement 5"() -> (w851:dbl[])
    n361 = case shown="\"Chien-Hrones-Reswick\"" "Control 5" {
      tunnel: w852 -> [w861 w869 w878 w887]
      tunnel: w851 -> [w860 w868 w877 w886]
      tunnel: [w859 w867 w876 w885] -> w839
      tunnel: [w858 w866 w875 w884] -> w838
      tunnel: w840 -> [w857 w865 w874 w883]
      tunnel: [w856 w864 w873 w882] -> w837
      tunnel: [w855 w863 w872 w881] -> w842
      tunnel: "Type of controller 5" -> [w854 w862 w871 w880]
      frame "Ziegler-Nichols", Default {
        n362 = call-poly <vilib>:"PID Autotuning Design.vi"("Ziegler-Nichols Speed"="Ziegler-Nichols speed 5", "Type of Controller"=w854, "dt (s)"=w857, "Response signal"=w860, "Stimulus signal"=w861) -> ("PID gains"=w855:T2, "response operating point"=w858:dbl, "stimulus operating point"=w859:dbl, "Plant Parameters"=w856:T4)  [unwired: 3 in]
      }
      frame "Cohen-Coon" {
        n363 = call-poly <vilib>:"PID Autotuning Design.vi"("Type of Controller"=w862, "dt (s)"=w865, "Response signal"=w868, "Stimulus signal"=w869) -> ("PID gains"=w863:T2, "response offset"=w866:dbl, "stimulus offset"=w867:dbl, "Plant Parameters"=w864:T4)  [unwired: 4 in]
      }
      frame "Chien-Hrones-Reswick" {
        n364 = call-poly <vilib>:"PID Autotuning Design.vi"("Tuning specifications"="Tuning specifications 5", "Type of Controller"=w871, "dt (s)"=w874, "Response signal"=w877, "Stimulus signal"=w878) -> ("PID gains"=w872:T2, "response offset"=w875:dbl, "stimulus offset"=w876:dbl, "Plant Parameters"=w873:T4)  [unwired: 3 in]
      }
      frame "Internal Model Control" {
        n365 = call-poly <vilib>:"PID Autotuning Design.vi"("Desired Time Constant (tau_c)"="Multiplicative factor 5", "Type of Controller"=w880, "dt (s)"=w883, "Response signal"=w886, "Stimulus signal"=w887) -> ("PID gains"=w881:T2, "response offset"=w884:dbl, "stimulus offset"=w885:dbl, "Plant Parameters"=w882:T4)  [unwired: 3 in]
      }
    }
    "Stimulus operating point 5" <- w839
    "Response operating point 5" <- w838
    "Identified Plant Parameters 5" <- w837
    n366 = Unbundle(w842) -> ("proportional gain (Kc)"=w845:dbl)  [unwired: 2 out]
    n367 = Equal?(x=w845, y=inf) -> (x = y?=w844:bool)
    n368 = feedback #16() -> (w843:T2)  [unwired: 1 in]
    n369 = Select(t=w843, s=w844, f=w842) -> (s? t:f=w841:T2)
    "Tuned PID gains 5" <- w841
    n370 = feedback-in #16(w841) -> ()
    n371 = case shown="True" "Accept gain 5" {
      tunnel: w841 -> [_ w888]
      frame False {
      }
      frame True {
        n372 = local write "PID Gains 5"(w888) -> ()
      }
    }
    n373 = local read "Stop 5"() -> (w850:bool)
  }
  n374 = while {
    tunnel: w79 -> [_]
    tunnel: w75 -> [w892]
    stop <- w902 stop-if-true
    # "If dT and deadtime have similar values, the identification could evaluate deadtime as zero and this generates proportional gain equal to Inf. This code avoid gain changes in this situations."
    # "Autotuning Loop"
    n375 = local read "Control Output 2"() -> (w904:dbl[])
    n376 = local read "Measurement 2"() -> (w903:dbl[])
    n377 = case shown="\"Chien-Hrones-Reswick\"" "Control 2" {
      tunnel: w904 -> [w913 w921 w930 w939]
      tunnel: w903 -> [w912 w920 w929 w938]
      tunnel: [w911 w919 w928 w937] -> w891
      tunnel: [w910 w918 w927 w936] -> w890
      tunnel: w892 -> [w909 w917 w926 w935]
      tunnel: [w908 w916 w925 w934] -> w889
      tunnel: [w907 w915 w924 w933] -> w894
      tunnel: "Type of controller 2" -> [w906 w914 w923 w932]
      frame "Ziegler-Nichols", Default {
        n378 = call-poly <vilib>:"PID Autotuning Design.vi"("Ziegler-Nichols Speed"="Ziegler-Nichols speed 2", "Type of Controller"=w906, "dt (s)"=w909, "Response signal"=w912, "Stimulus signal"=w913) -> ("PID gains"=w907:T2, "response operating point"=w910:dbl, "stimulus operating point"=w911:dbl, "Plant Parameters"=w908:T4)  [unwired: 3 in]
      }
      frame "Cohen-Coon" {
        n379 = call-poly <vilib>:"PID Autotuning Design.vi"("Type of Controller"=w914, "dt (s)"=w917, "Response signal"=w920, "Stimulus signal"=w921) -> ("PID gains"=w915:T2, "response offset"=w918:dbl, "stimulus offset"=w919:dbl, "Plant Parameters"=w916:T4)  [unwired: 4 in]
      }
      frame "Chien-Hrones-Reswick" {
        n380 = call-poly <vilib>:"PID Autotuning Design.vi"("Tuning specifications"="Tuning specifications 2", "Type of Controller"=w923, "dt (s)"=w926, "Response signal"=w929, "Stimulus signal"=w930) -> ("PID gains"=w924:T2, "response offset"=w927:dbl, "stimulus offset"=w928:dbl, "Plant Parameters"=w925:T4)  [unwired: 3 in]
      }
      frame "Internal Model Control" {
        n381 = call-poly <vilib>:"PID Autotuning Design.vi"("Desired Time Constant (tau_c)"="Multiplicative factor 2", "Type of Controller"=w932, "dt (s)"=w935, "Response signal"=w938, "Stimulus signal"=w939) -> ("PID gains"=w933:T2, "response offset"=w936:dbl, "stimulus offset"=w937:dbl, "Plant Parameters"=w934:T4)  [unwired: 3 in]
      }
    }
    "Stimulus operating point 2" <- w891
    "Response operating point 2" <- w890
    "Identified Plant Parameters 2" <- w889
    n382 = Unbundle(w894) -> ("proportional gain (Kc)"=w897:dbl)  [unwired: 2 out]
    n383 = Equal?(x=w897, y=inf) -> (x = y?=w896:bool)
    n384 = feedback #17() -> (w895:T2)  [unwired: 1 in]
    n385 = Select(t=w895, s=w896, f=w894) -> (s? t:f=w893:T2)
    "Tuned PID gains 2" <- w893
    n386 = feedback-in #17(w893) -> ()
    n387 = case shown="True" "Accept gain 2" {
      tunnel: w893 -> [_ w940]
      frame False {
      }
      frame True {
        n388 = local write "PID Gains 2"(w940) -> ()
      }
    }
    n389 = local read "Stop 2"() -> (w902:bool)
  }
  n390 = while {
    tunnel: w121 -> [_]
    tunnel: w117 -> [w944]
    stop <- w954 stop-if-true
    # "If dT and deadtime have similar values, the identification could evaluate deadtime as zero and this generates proportional gain equal to Inf. This code avoid gain changes in this situations."
    # "Autotuning Loop"
    n391 = local read "Control Output"() -> (w956:dbl[])
    n392 = local read "Measurement"() -> (w955:dbl[])
    n393 = case shown="\"Chien-Hrones-Reswick\"" "Control" {
      tunnel: w956 -> [w965 w973 w982 w991]
      tunnel: w955 -> [w964 w972 w981 w990]
      tunnel: [w963 w971 w980 w989] -> w943
      tunnel: [w962 w970 w979 w988] -> w942
      tunnel: w944 -> [w961 w969 w978 w987]
      tunnel: [w960 w968 w977 w986] -> w941
      tunnel: [w959 w967 w976 w985] -> w946
      tunnel: "Type of controller" -> [w958 w966 w975 w984]
      frame "Ziegler-Nichols", Default {
        n394 = call-poly <vilib>:"PID Autotuning Design.vi"("Ziegler-Nichols Speed"="Ziegler-Nichols speed", "Type of Controller"=w958, "dt (s)"=w961, "Response signal"=w964, "Stimulus signal"=w965) -> ("PID gains"=w959:T2, "response operating point"=w962:dbl, "stimulus operating point"=w963:dbl, "Plant Parameters"=w960:T4)  [unwired: 3 in]
      }
      frame "Cohen-Coon" {
        n395 = call-poly <vilib>:"PID Autotuning Design.vi"("Type of Controller"=w966, "dt (s)"=w969, "Response signal"=w972, "Stimulus signal"=w973) -> ("PID gains"=w967:T2, "response offset"=w970:dbl, "stimulus offset"=w971:dbl, "Plant Parameters"=w968:T4)  [unwired: 4 in]
      }
      frame "Chien-Hrones-Reswick" {
        n396 = call-poly <vilib>:"PID Autotuning Design.vi"("Tuning specifications"="Tuning specifications", "Type of Controller"=w975, "dt (s)"=w978, "Response signal"=w981, "Stimulus signal"=w982) -> ("PID gains"=w976:T2, "response offset"=w979:dbl, "stimulus offset"=w980:dbl, "Plant Parameters"=w977:T4)  [unwired: 3 in]
      }
      frame "Internal Model Control" {
        n397 = call-poly <vilib>:"PID Autotuning Design.vi"("Desired Time Constant (tau_c)"="Multiplicative factor", "Type of Controller"=w984, "dt (s)"=w987, "Response signal"=w990, "Stimulus signal"=w991) -> ("PID gains"=w985:T2, "response offset"=w988:dbl, "stimulus offset"=w989:dbl, "Plant Parameters"=w986:T4)  [unwired: 3 in]
      }
    }
    "Stimulus operating point" <- w943
    "Response operating point" <- w942
    "Identified Plant Parameters" <- w941
    n398 = Unbundle(w946) -> ("proportional gain (Kc)"=w949:dbl)  [unwired: 2 out]
    n399 = Equal?(x=w949, y=inf) -> (x = y?=w948:bool)
    n400 = feedback #18() -> (w947:T2)  [unwired: 1 in]
    n401 = Select(t=w947, s=w948, f=w946) -> (s? t:f=w945:T2)
    "Tuned PID gains" <- w945
    n402 = feedback-in #18(w945) -> ()
    n403 = case shown="True" "Accept gain" {
      tunnel: w945 -> [_ w992]
      frame False {
      }
      frame True {
        n404 = local write "PID Gains"(w992) -> ()
      }
    }
    n405 = local read "Stop"() -> (w954:bool)
  }
  n406 = while {
    shift-right: [w1000] -> w113
    shift-left: w112 -> [w996]
    tunnel: w111 -> [w995]
    tunnel: [w997] -> w114
    stop <- w998 stop-if-true
    # "Serial Read Loop"
    n407 = case shown="True" TRUE {
      tunnel: [w1012 w1016] -> w1000
      tunnel: w996 -> [w1014 w1016]
      tunnel: [w1011 w1015] -> w997
      tunnel: w995 -> [w1013 w1015]
      frame True {
        n408 = VISA Read(VISA resource name=w1014, byte count=u32 1000, error in (no error)=w1013) -> (VISA resource name out=w1012:refnum<visa-resource-name>, read buffer=w1009:string, error out=w1011:errorcluster)  [unwired: 1 out]
        n409 = Decimal String To Number(string=w1009) -> (number=w1007:i32)  [unwired: 2 in, 1 out]
        "Sensor Raw Value" <- w1007
        n410 = call <vilib>:"Median PtByPt.vi"("sample length"=20, "x"=w1007) -> ("median"=w1005:dbl)  [unwired: 2 in, 1 out]
        n411 = To Double Precision Float(number=w1005) -> (double precision float=w1001:dbl)
        n412 = Multiply(x=w1001, y=0.0292) -> (x*y=w1004:dbl)
        "Force in Kilograms 2" <- w1004
        n413 = Multiply(x=w1004, y=9.81) -> (x*y=→"Force in Newtons 2":dbl)
      }
      frame False {
      }
    }
    n414 = Wait (ms)(milliseconds to wait=u32 5) -> ()  [unwired: 1 out]
    n415 = Or(x=w997, y=FALSE) -> (x .or. y?=w998:bool)
  }
  n416 = while {
    shift-right: [w1024] -> w81
    shift-left: w107 -> [w1020]
    tunnel: w106 -> [w1019]
    tunnel: [w1021] -> w108
    stop <- w1022 stop-if-true
    # "Serial Read Loop"
    n417 = case shown="True" TRUE {
      tunnel: [w1036 w1040] -> w1024
      tunnel: w1020 -> [w1038 w1040]
      tunnel: [w1035 w1039] -> w1021
      tunnel: w1019 -> [w1037 w1039]
      frame True {
        n418 = VISA Read(VISA resource name=w1038, byte count=u32 1000, error in (no error)=w1037) -> (VISA resource name out=w1036:refnum<visa-resource-name>, read buffer=w1033:string, error out=w1035:errorcluster)  [unwired: 1 out]
        n419 = Decimal String To Number(string=w1033) -> (number=w1029:i32)  [unwired: 2 in, 1 out]
        "Sensor Raw Value 2" <- w1029
        n420 = call <vilib>:"Median PtByPt.vi"("sample length"=20, "x"=w1029) -> ("median"=w1030:dbl)  [unwired: 2 in, 1 out]
        n421 = To Double Precision Float(number=w1030) -> (double precision float=w1026:dbl)
        n422 = Multiply(x=w1026, y=0.0238) -> (x*y=w1025:dbl)
        "Force in Kilograms" <- w1025
        n423 = Multiply(x=w1025, y=9.81) -> (x*y=→"Force in Newtons":dbl)
      }
      frame False {
      }
    }
    n424 = Or(x=w1021, y=FALSE) -> (x .or. y?=w1022:bool)
    n425 = Wait (ms)(milliseconds to wait=u32 5) -> ()  [unwired: 1 out]
  }
  n426 = VISA Close(VISA resource name=w113, error in (no error)=w114) -> (error out=w115:errorcluster)
  n427 = call <vilib>:"Simple Error Handler.vi"("error in (no error)"=w115) -> ()  [unwired: 1 in, 8 out]
  n428 = VISA Close(VISA resource name=w81, error in (no error)=w108) -> (error out=w109:errorcluster)
  n429 = call <vilib>:"Simple Error Handler.vi"("error in (no error)"=w109) -> ()  [unwired: 1 in, 8 out]
  n430 = stacked-sequence {
    tunnel: [_ w1046] -> w88
    tunnel: [_ w1045] -> w87
    frame #0 {
      w1041 = 0
      w1042 = FALSE
      w1043 = ""
      # "Initialize Indicators"
      "Connected" <- w1042
      "Start Time Text" <- w1043
      "Stop Time Text" <- w1043
      "Elapsed Time Text" <- w1043
      "HostFrameCount" <- w1041
      "Running" <- w1042
      "Loop Iter" <- w1041
      "PnoData" <- w1042
    }
    frame #1 {
      # "Connect To Tracker"
      # "2. Initialize Tracker Connection"
      n431 = call <instrlib>:"PDI initialize.vi"() -> ("error out"=w1045:errorcluster, "Connected"=w1044:bool, "pDev"=w1046:u32)  [unwired: 1 in, 4 out]
      n432 = local write "Connected"(w1044) -> ()
    }
  }
  n433 = while {
    stop <- FALSE stop-if-true
    # "TRACKER 4"
    # "TRACKER 3"
    # "TRACKER 2"
    # "TRACKER 1"
    n434 = Index Array(array="XYZAER", index #1=0 ("index"), index #2=1 ("index"), index #3=2 ("index"), index #4=3 ("index")) -> (element #1=w1071:T8, element #2=w1070:T8, element #3=w1069:T8, element #4=w1068:T8)
    n435 = Unbundle By Name(w1071) -> ("x"=w1058:sgl, "y"=w1057:sgl)  [unwired: 1 out]
    n436 = Unbundle By Name(w1070) -> ("x"=w1055:sgl, "y"=w1054:sgl)  [unwired: 1 out]
    n437 = Multiply(x=w1057, y=sgl -1.0) -> (x*y=w1056:sgl)
    n438 = Multiply(x=w1054, y=-1.0) -> (x*y=w1053:dbl)
    n439 = Bundle(w1053, "x"=w1055) -> (w1066:cluster{dbl, "x":sgl})  [unwired: 1 in]
    n440 = Bundle(w1056, "x"=w1058) -> (w1067:cluster{sgl, "x":sgl})  [unwired: 1 in]
    n441 = Unbundle By Name(w1069) -> ("x"=w1052:sgl, "y"=w1051:sgl)  [unwired: 1 out]
    n442 = Unbundle By Name(w1068) -> ("x"=w1049:sgl, "y"=w1048:sgl)  [unwired: 1 out]
    n443 = Multiply(x=w1051, y=-1.0) -> (x*y=w1050:dbl)
    n444 = Multiply(x=w1048, y=-1.0) -> (x*y=w1047:dbl)
    n445 = Bundle(w1050, "x"=w1052) -> (w1065:cluster{dbl, "x":sgl})  [unwired: 1 in]
    n446 = Bundle(w1047, "x"=w1049) -> (w1064:cluster{dbl, "x":sgl})  [unwired: 1 in]
    n447 = Build Array(w1067, w1066, w1065, w1064) -> (→"Position Sensor Data":cluster{dbl, "x":sgl}[])
  }
  n448 = call <instrlib>:"PDI util stationcount.vi"("error in (no error)"=w87, "pDev"=w88) -> ("error out"=w86:errorcluster, "dup pDev"=w85:u32, "MaxCount"=w83:i32)  [unwired: 7 out]
  n449 = call <instrlib>:"PDI config setbuffer.vi"("error in (no error)"=w86, "Max sensors"=w83, "FrameCount"=w84, "pDev"=w85) -> ("error out"=w95:errorcluster, "dup pDev"=w96:u32)  [unwired: 6 out]
  n450 = flat-sequence {
    tunnel: w101 -> [_]
    tunnel: [w1078] -> w97
    frame #0 {
      # "Get Start Time"
      n451 = Get Date/Time In Seconds() -> (seconds since 1Jan1904=w1079:timestamp)
      n452 = Format Date/Time String(seconds (now)=w1079) -> (date/time string=w1080:string)  [unwired: 2 out]
      n453 = local write "Start Time Text"(w1080) -> ()
      n454 = To Double Precision Float(number=w1079) -> (double precision float=w1078:dbl)
    }
  }
  n455 = call <instrlib>:"PDI action startcont.vi"("error in (no error)"=w95, "pDev"=w96) -> ("error out"=w102:errorcluster, "Running"=w94:bool, "dup pDev"=w101:u32)  [unwired: 7 out]
  n456 = control-ref of="HostFrameCount"() -> (w92:refnum<vi>)
  n457 = local write "Running"(w94) -> ()
  n458 = while {
    shift-left: 0.0 ("Plant Output") -> [w1146]
    shift-right: [w1141] -> _
    tunnel: w25 -> [_]
    shift-right: [w1127] -> _
    shift-left: 0.01 -> [w1125]
    shift-right: [w1099] -> _
    shift-left: TRUE -> [w1124]
    shift-right: [w1101] -> _
    shift-left: w22 -> [w1123]
    shift-right: [w1126] -> _
    shift-left: w22 -> [w1122]
    tunnel: [w1096] -> w21
    tunnel: w14 -> [w1082]
    tunnel: [w1081] -> w5
    stop <- "Stop 11" stop-if-true
    w1087 = 1 items=["one channel for each line", "one channel for all lines"] ("line grouping")
    w1096 = 0.05 ("Sampling Time dt (s)")
    w1105 = 1 items=["one channel for each line", "one channel for all lines"] ("line grouping")
    w1113 = 0.5 ("x")
    w1140 = T7 {"static gain"=2.5, "lag (s)"=2.5, "deadtime (s)"=0.01, "load"=0.0, "deadband"=0.0, "sensor noise"=0.0, "initial PV"=30.0, "plant noise"=0.0}  # Process parameters
    w1142 = FALSE  # Integrator ?
    # "C."
    # "Inlet 11"
    # "Exhaust 5"
    # "B."
    # "A."
    # "A.Output to PWM Logic \nB. Simulated Plant\nC. Draw Chart"
    # "Main PID Loop Control"
    n459 = Multiply(x=w1096, y=1000.0) -> (x*y=w1139:dbl)
    n460 = Not(x="Autotune 11") -> (.not. x?=w1143:bool)
    n461 = feedback #19() -> (w1148:bool)  [unwired: 1 in]
    n462 = feedback-in #19("Autotune 11") -> ()
    n463 = Wait Until Next ms Multiple(millisecond multiple=w1139) -> ()  [unwired: 1 out]
    n464 = Exclusive Or(1:w1148, 2:"Autotune 11") -> (0:w1147:bool)
    n465 = feedback #20() -> (w1145:dbl)  [unwired: 1 in]
    n466 = Multiply(x=w1082, y=-1000.0) -> (x*y=w1129:dynamicdata)
    n467 = call <vilib>:"Median PtByPt.vi"("sample length"="Median sample length 20", "x"=w1129) -> ("median"=w1128:dbl)  [unwired: 2 in, 1 out]
    n468 = Square(x=w1128) -> (x^2=w1136:dbl)
    n469 = Multiply(x=w1128, y=-39.646) -> (x*y=w1132:dbl)
    n470 = Multiply(x=w1136, y=0.2324) -> (x*y=w1133:dbl)
    n471 = Add(x=w1132, y=w1133) -> (x+y=w1131:dbl)
    n472 = Add(x=1678.0, y=w1131) -> (x+y=w1094:dbl)
    n473 = case shown="False" "Autotune 11" {
      tunnel: w1096 -> [w1163 _]
      tunnel: [w1152 w1168] -> w1101
      tunnel: w1146 -> [_ w1167]
      tunnel: "PID Gains 11" -> [w1162 _]
      tunnel: "Reinitialize 11" -> [w1159 _]
      tunnel: w1147 -> [w1161 w1166]
      tunnel: w1145 -> [_ w1170]
      tunnel: w1094 -> [w1155 _]
      tunnel: "Set Point 11" -> [w1154 _]
      frame False {
        # "This code is to have 'bumpless' transfer from autotuning"
        n474 = Not(x=w1161) -> (.not. x?=w1158:bool)
        n475 = And(x="Automatic 11", y=w1158) -> (x .and. y?=w1160:bool)
        n476 = call-poly <vilib>:"PID Advanced.vi"("setpoint"=w1154, "auto? (T)"=w1160, "manual control"="MV: 11", "process variable"=w1155, "alpha"=10.0, "PID gains"=w1162, "dt (s)"=w1163, "reinitialize? (F)"=w1159) -> ("output"=w1152:dbl)  [unwired: 6 in, 1 out]
      }
      frame True {
        w1173 = 10000 ("sample length")
        # "Buffering data for parameters estimation"
        n477 = call <vilib>:"Data Queue PtByPt.vi"("initial queue element"=w1167, "initialize"=w1166, "sample length"=w1173, "input data point"=w1167) -> ("Current Queue"=→"Control Output 11":dbl[])  [unwired: 3 in, 4 out]
        n478 = Select(t=0.0, s=w1166, f="Excitation 11") -> (s? t:f=w1171:dbl)
        n479 = Add(x=w1170, y=w1171) -> (x+y=w1168:dbl)
        n480 = call <vilib>:"Data Queue PtByPt.vi"("initial queue element"=w1168, "initialize"=w1166, "sample length"=w1173, "input data point"=w1168) -> ("Current Queue"=→"Measurement 11":dbl[])  [unwired: 3 in, 4 out]
      }
    }
    n481 = feedback-in #20(w1101, w1143) -> ()
    n482 = Greater?(x=w1094, y="M-5") -> (0:w1081:bool)
    n483 = Add(x=w1125, y=w1113) -> (x+y=w1114:dbl)
    n484 = Subtract(x=w1125, y=w1113) -> (x-y=w1112:dbl)
    n485 = Equal?(x=w1123, y=w1101) -> (x = y?=w1120:bool)
    n486 = Greater?(x=w1101, y=w1123) -> (0:w1119:bool)
    n487 = Select(t=w1124, s=w1120, f=w1119) -> (s? t:f=w1099:bool)
    "PWM Output 11" <- w1099
    n488 = call "Plant System.vi"("Integrator ?"=w1142, "Plant Input"=w1101, "dt (s)"=w1096, "process parameters"=w1140) -> ("Plant Output"=w1141:dbl)  [unwired: 11 in]
    n489 = Increment(x="Set Point 11") -> (x+1=w1118:dbl)
    n490 = Decrement(x="Set Point 11") -> (x-1=w1117:dbl)
    n491 = Select(t=w1114, s=w1099, f=w1112) -> (s? t:f=w1127:dbl)
    n492 = Select(t=w1118, s=w1099, f=w1117) -> (s? t:f=w1116:dbl)
    n493 = Not(x=w1099) -> (.not. x?=w1098:bool)
    n494 = call-poly <vilib>:"DAQmx Create Virtual Channel.vi"("lines"=tag "cDAQ1Mod1/port0/line5", "line grouping"=w1105) -> ("task out"=w1107:refnum<k21>, "error out"=w1106:errorcluster)  [unwired: 12 in]
    n495 = call-poly <vilib>:"DAQmx Create Virtual Channel.vi"("lines"=tag "cDAQ1Mod2/port0/line5", "line grouping"=w1087) -> ("task out"=w1089:refnum<k21>, "error out"=w1088:errorcluster)  [unwired: 12 in]
    n496 = Build Array(w1094, "Set Point 11", w1116) -> (w1115:dbl[])
    n497 = Initialize Array("INLET 5 ON/OFF 3", 1 ("dimension size")) -> (w1084:bool[])
    n498 = Initialize Array(w1098, 1 ("dimension size")) -> (w1102:bool[])
    n499 = local write "MV: 11"(w1101) -> ()
    n500 = Add(x=w1122, y=w1125) -> (x+y=w1126:dbl)
    n501 = Build Array(w1115) -> (→"Real time Data 11":dbl[][])
    n502 = call-poly <vilib>:"DAQmx Write.vi"("task/channels in"=w1107, "auto start"=TRUE, "data"=w1102, "error in"=w1106) -> ("task out"=w1109:refnum<k21>, "error out"=w1110:errorcluster)  [unwired: 9 in, 1 out]
    n503 = call-poly <vilib>:"DAQmx Write.vi"("task/channels in"=w1089, "auto start"=TRUE, "data"=w1084, "error in"=w1088) -> ("task out"=w1091:refnum<k21>, "error out"=w1092:errorcluster)  [unwired: 9 in, 1 out]
    n504 = call <vilib>:"DAQmx Clear Task.vi"("task in"=w1109, "error in"=w1110) -> ("error out"=w1104:errorcluster)  [unwired: 13 in]
    n505 = call <vilib>:"DAQmx Clear Task.vi"("task in"=w1091, "error in"=w1092) -> ("error out"=w1086:errorcluster)  [unwired: 13 in]
    n506 = call <vilib>:"Simple Error Handler.vi"("error in (no error)"=w1104) -> ()  [unwired: 4 in, 5 out]
    n507 = call <vilib>:"Simple Error Handler.vi"("error in (no error)"=w1086) -> ()  [unwired: 4 in, 5 out]
  }
  n508 = while {
    shift-left: 0.0 ("Plant Output") -> [w1239]
    shift-right: [w1234] -> _
    tunnel: w19 -> [_]
    shift-right: [w1220] -> _
    shift-left: 0.01 -> [w1218]
    shift-right: [w1192] -> _
    shift-left: TRUE -> [w1217]
    shift-right: [w1194] -> _
    shift-left: w16 -> [w1216]
    shift-right: [w1219] -> _
    shift-left: w16 -> [w1215]
    tunnel: [w1189] -> w15
    tunnel: w14 -> [w1175]
    tunnel: [w1174] -> w6
    stop <- "Stop 12" stop-if-true
    w1180 = 1 items=["one channel for each line", "one channel for all lines"] ("line grouping")
    w1189 = 0.05 ("Sampling Time dt (s)")
    w1198 = 1 items=["one channel for each line", "one channel for all lines"] ("line grouping")
    w1206 = 0.5 ("x")
    w1233 = T7 {"static gain"=2.5, "lag (s)"=2.5, "deadtime (s)"=0.01, "load"=0.0, "deadband"=0.0, "sensor noise"=0.0, "initial PV"=30.0, "plant noise"=0.0}  # Process parameters
    w1235 = FALSE  # Integrator ?
    # "C."
    # "Inlet 11"
    # "Exhaust 1"
    # "B."
    # "A."
    # "A.Output to PWM Logic \nB. Simulated Plant\nC. Draw Chart"
    # "Main PID Loop Control"
    n509 = Multiply(x=w1189, y=1000.0) -> (x*y=w1232:dbl)
    n510 = Not(x="Autotune 12") -> (.not. x?=w1236:bool)
    n511 = feedback #21() -> (w1241:bool)  [unwired: 1 in]
    n512 = feedback-in #21("Autotune 12") -> ()
    n513 = Wait Until Next ms Multiple(millisecond multiple=w1232) -> ()  [unwired: 1 out]
    n514 = Exclusive Or(1:w1241, 2:"Autotune 12") -> (0:w1240:bool)
    n515 = feedback #22() -> (w1238:dbl)  [unwired: 1 in]
    n516 = Multiply(x=w1175, y=-1000.0) -> (x*y=w1222:dynamicdata)
    n517 = call <vilib>:"Median PtByPt.vi"("sample length"="Median sample length 21", "x"=w1222) -> ("median"=w1221:dbl)  [unwired: 2 in, 1 out]
    n518 = Square(x=w1221) -> (x^2=w1229:dbl)
    n519 = Multiply(x=w1221, y=-39.646) -> (x*y=w1225:dbl)
    n520 = Multiply(x=w1229, y=0.2324) -> (x*y=w1226:dbl)
    n521 = Add(x=w1225, y=w1226) -> (x+y=w1224:dbl)
    n522 = Add(x=1678.0, y=w1224) -> (x+y=w1187:dbl)
    n523 = case shown="False" "Autotune 12" {
      tunnel: w1189 -> [w1256 _]
      tunnel: [w1245 w1261] -> w1194
      tunnel: w1239 -> [_ w1260]
      tunnel: "PID Gains 12" -> [w1255 _]
      tunnel: "Reinitialize 12" -> [w1252 _]
      tunnel: w1240 -> [w1254 w1259]
      tunnel: w1238 -> [_ w1263]
      tunnel: w1187 -> [w1248 _]
      tunnel: "Set Point 12" -> [w1247 _]
      frame False {
        # "This code is to have 'bumpless' transfer from autotuning"
        n524 = Not(x=w1254) -> (.not. x?=w1251:bool)
        n525 = And(x="Automatic 12", y=w1251) -> (x .and. y?=w1253:bool)
        n526 = call-poly <vilib>:"PID Advanced.vi"("setpoint"=w1247, "auto? (T)"=w1253, "manual control"="MV: 12", "process variable"=w1248, "alpha"=10.0, "PID gains"=w1255, "dt (s)"=w1256, "reinitialize? (F)"=w1252) -> ("output"=w1245:dbl)  [unwired: 6 in, 1 out]
      }
      frame True {
        w1266 = 10000 ("sample length")
        # "Buffering data for parameters estimation"
        n527 = call <vilib>:"Data Queue PtByPt.vi"("initial queue element"=w1260, "initialize"=w1259, "sample length"=w1266, "input data point"=w1260) -> ("Current Queue"=→"Control Output 12":dbl[])  [unwired: 3 in, 4 out]
        n528 = Select(t=0.0, s=w1259, f="Excitation 12") -> (s? t:f=w1264:dbl)
        n529 = Add(x=w1263, y=w1264) -> (x+y=w1261:dbl)
        n530 = call <vilib>:"Data Queue PtByPt.vi"("initial queue element"=w1261, "initialize"=w1259, "sample length"=w1266, "input data point"=w1261) -> ("Current Queue"=→"Measurement 12":dbl[])  [unwired: 3 in, 4 out]
      }
    }
    n531 = feedback-in #22(w1194, w1236) -> ()
    n532 = Greater?(x=w1187, y="M-1") -> (0:w1174:bool)
    n533 = Add(x=w1218, y=w1206) -> (x+y=w1207:dbl)
    n534 = Subtract(x=w1218, y=w1206) -> (x-y=w1205:dbl)
    n535 = Equal?(x=w1216, y=w1194) -> (x = y?=w1213:bool)
    n536 = Greater?(x=w1194, y=w1216) -> (0:w1212:bool)
    n537 = Select(t=w1217, s=w1213, f=w1212) -> (s? t:f=w1192:bool)
    "PWM Output 12" <- w1192
    n538 = call "Plant System.vi"("Integrator ?"=w1235, "Plant Input"=w1194, "dt (s)"=w1189, "process parameters"=w1233) -> ("Plant Output"=w1234:dbl)  [unwired: 11 in]
    n539 = Increment(x="Set Point 12") -> (x+1=w1211:dbl)
    n540 = Decrement(x="Set Point 12") -> (x-1=w1210:dbl)
    n541 = Select(t=w1207, s=w1192, f=w1205) -> (s? t:f=w1220:dbl)
    n542 = Select(t=w1211, s=w1192, f=w1210) -> (s? t:f=w1209:dbl)
    n543 = Not(x=w1192) -> (.not. x?=w1191:bool)
    n544 = call-poly <vilib>:"DAQmx Create Virtual Channel.vi"("lines"=tag "cDAQ1Mod1/port0/line7", "line grouping"=w1198) -> ("task out"=w1200:refnum<k21>, "error out"=w1199:errorcluster)  [unwired: 12 in]
    n545 = call-poly <vilib>:"DAQmx Create Virtual Channel.vi"("lines"=tag "cDAQ1Mod2/port0/line7", "line grouping"=w1180) -> ("task out"=w1182:refnum<k21>, "error out"=w1181:errorcluster)  [unwired: 12 in]
    n546 = Build Array(w1187, "Set Point 12", w1209) -> (w1208:dbl[])
    n547 = Initialize Array("INLET 1 ON/OFF 3", 1 ("dimension size")) -> (w1177:bool[])
    n548 = Initialize Array(w1191, 1 ("dimension size")) -> (w1195:bool[])
    n549 = local write "MV: 12"(w1194) -> ()
    n550 = Add(x=w1215, y=w1218) -> (x+y=w1219:dbl)
    n551 = Build Array(w1208) -> (→"Real time Data 12":dbl[][])
    n552 = call-poly <vilib>:"DAQmx Write.vi"("task/channels in"=w1200, "auto start"=TRUE, "data"=w1195, "error in"=w1199) -> ("task out"=w1202:refnum<k21>, "error out"=w1203:errorcluster)  [unwired: 9 in, 1 out]
    n553 = call-poly <vilib>:"DAQmx Write.vi"("task/channels in"=w1182, "auto start"=TRUE, "data"=w1177, "error in"=w1181) -> ("task out"=w1184:refnum<k21>, "error out"=w1185:errorcluster)  [unwired: 9 in, 1 out]
    n554 = call <vilib>:"DAQmx Clear Task.vi"("task in"=w1202, "error in"=w1203) -> ("error out"=w1197:errorcluster)  [unwired: 13 in]
    n555 = call <vilib>:"DAQmx Clear Task.vi"("task in"=w1184, "error in"=w1185) -> ("error out"=w1179:errorcluster)  [unwired: 13 in]
    n556 = call <vilib>:"Simple Error Handler.vi"("error in (no error)"=w1197) -> ()  [unwired: 4 in, 5 out]
    n557 = call <vilib>:"Simple Error Handler.vi"("error in (no error)"=w1179) -> ()  [unwired: 4 in, 5 out]
  }
  n558 = while {
    shift-left: 0.0 ("Plant Output") -> [w1332]
    shift-right: [w1327] -> _
    tunnel: w31 -> [_]
    shift-right: [w1313] -> _
    shift-left: 0.01 -> [w1311]
    shift-right: [w1285] -> _
    shift-left: TRUE -> [w1310]
    shift-right: [w1287] -> _
    shift-left: w28 -> [w1309]
    shift-right: [w1312] -> _
    shift-left: w28 -> [w1308]
    tunnel: [w1282] -> w27
    tunnel: w14 -> [w1268]
    tunnel: [w1267] -> w4
    stop <- "Stop 10" stop-if-true
    w1273 = 1 items=["one channel for each line", "one channel for all lines"] ("line grouping")
    w1282 = 0.05 ("Sampling Time dt (s)")
    w1291 = 1 items=["one channel for each line", "one channel for all lines"] ("line grouping")
    w1299 = 0.5 ("x")
    w1326 = T7 {"static gain"=2.5, "lag (s)"=2.5, "deadtime (s)"=0.01, "load"=0.0, "deadband"=0.0, "sensor noise"=0.0, "initial PV"=30.0, "plant noise"=0.0}  # Process parameters
    w1328 = FALSE  # Integrator ?
    # "C."
    # "Inlet 11"
    # "Exhaust 3"
    # "B."
    # "A."
    # "A.Output to PWM Logic \nB. Simulated Plant\nC. Draw Chart"
    # "Main PID Loop Control"
    n559 = Multiply(x=w1282, y=1000.0) -> (x*y=w1325:dbl)
    n560 = Not(x="Autotune 10") -> (.not. x?=w1329:bool)
    n561 = feedback #23() -> (w1334:bool)  [unwired: 1 in]
    n562 = feedback-in #23("Autotune 10") -> ()
    n563 = Wait Until Next ms Multiple(millisecond multiple=w1325) -> ()  [unwired: 1 out]
    n564 = Exclusive Or(1:w1334, 2:"Autotune 10") -> (0:w1333:bool)
    n565 = feedback #24() -> (w1331:dbl)  [unwired: 1 in]
    n566 = Multiply(x=w1268, y=-1000.0) -> (x*y=w1315:dynamicdata)
    n567 = call <vilib>:"Median PtByPt.vi"("sample length"="Median sample length 19", "x"=w1315) -> ("median"=w1314:dbl)  [unwired: 2 in, 1 out]
    n568 = Square(x=w1314) -> (x^2=w1322:dbl)
    n569 = Multiply(x=w1314, y=-39.646) -> (x*y=w1318:dbl)
    n570 = Multiply(x=w1322, y=0.2324) -> (x*y=w1319:dbl)
    n571 = Add(x=w1318, y=w1319) -> (x+y=w1317:dbl)
    n572 = Add(x=1678.0, y=w1317) -> (x+y=w1280:dbl)
    n573 = case shown="False" "Autotune 10" {
      tunnel: w1282 -> [w1349 _]
      tunnel: [w1338 w1354] -> w1287
      tunnel: w1332 -> [_ w1353]
      tunnel: "PID Gains 10" -> [w1348 _]
      tunnel: "Reinitialize 10" -> [w1345 _]
      tunnel: w1333 -> [w1347 w1352]
      tunnel: w1331 -> [_ w1356]
      tunnel: w1280 -> [w1341 _]
      tunnel: "Set Point 10" -> [w1340 _]
      frame False {
        # "This code is to have 'bumpless' transfer from autotuning"
        n574 = Not(x=w1347) -> (.not. x?=w1344:bool)
        n575 = And(x="Automatic 10", y=w1344) -> (x .and. y?=w1346:bool)
        n576 = call-poly <vilib>:"PID Advanced.vi"("setpoint"=w1340, "auto? (T)"=w1346, "manual control"="MV: 10", "process variable"=w1341, "alpha"=10.0, "PID gains"=w1348, "dt (s)"=w1349, "reinitialize? (F)"=w1345) -> ("output"=w1338:dbl)  [unwired: 6 in, 1 out]
      }
      frame True {
        w1359 = 10000 ("sample length")
        # "Buffering data for parameters estimation"
        n577 = call <vilib>:"Data Queue PtByPt.vi"("initial queue element"=w1353, "initialize"=w1352, "sample length"=w1359, "input data point"=w1353) -> ("Current Queue"=→"Control Output 10":dbl[])  [unwired: 3 in, 4 out]
        n578 = Select(t=0.0, s=w1352, f="Excitation 10") -> (s? t:f=w1357:dbl)
        n579 = Add(x=w1356, y=w1357) -> (x+y=w1354:dbl)
        n580 = call <vilib>:"Data Queue PtByPt.vi"("initial queue element"=w1354, "initialize"=w1352, "sample length"=w1359, "input data point"=w1354) -> ("Current Queue"=→"Measurement 10":dbl[])  [unwired: 3 in, 4 out]
      }
    }
    n581 = feedback-in #24(w1287, w1329) -> ()
    n582 = Greater?(x=w1280, y="M-3") -> (0:w1267:bool)
    n583 = Add(x=w1311, y=w1299) -> (x+y=w1300:dbl)
    n584 = Subtract(x=w1311, y=w1299) -> (x-y=w1298:dbl)
    n585 = Equal?(x=w1309, y=w1287) -> (x = y?=w1306:bool)
    n586 = Greater?(x=w1287, y=w1309) -> (0:w1305:bool)
    n587 = Select(t=w1310, s=w1306, f=w1305) -> (s? t:f=w1285:bool)
    "PWM Output 10" <- w1285
    n588 = call "Plant System.vi"("Integrator ?"=w1328, "Plant Input"=w1287, "dt (s)"=w1282, "process parameters"=w1326) -> ("Plant Output"=w1327:dbl)  [unwired: 11 in]
    n589 = Increment(x="Set Point 10") -> (x+1=w1304:dbl)
    n590 = Decrement(x="Set Point 10") -> (x-1=w1303:dbl)
    n591 = Select(t=w1300, s=w1285, f=w1298) -> (s? t:f=w1313:dbl)
    n592 = Select(t=w1304, s=w1285, f=w1303) -> (s? t:f=w1302:dbl)
    n593 = Not(x=w1285) -> (.not. x?=w1284:bool)
    n594 = call-poly <vilib>:"DAQmx Create Virtual Channel.vi"("lines"=tag "cDAQ1Mod8/port0/line7", "line grouping"=w1291) -> ("task out"=w1293:refnum<k21>, "error out"=w1292:errorcluster)  [unwired: 12 in]
    n595 = call-poly <vilib>:"DAQmx Create Virtual Channel.vi"("lines"=tag "cDAQ1Mod7/port0/line6", "line grouping"=w1273) -> ("task out"=w1275:refnum<k21>, "error out"=w1274:errorcluster)  [unwired: 12 in]
    n596 = Build Array(w1280, "Set Point 10", w1302) -> (w1301:dbl[])
    n597 = Initialize Array("INLET 3 ON/OFF 3", 1 ("dimension size")) -> (w1270:bool[])
    n598 = Initialize Array(w1284, 1 ("dimension size")) -> (w1288:bool[])
    n599 = local write "MV: 10"(w1287) -> ()
    n600 = Add(x=w1308, y=w1311) -> (x+y=w1312:dbl)
    n601 = Build Array(w1301) -> (→"Real time Data 10":dbl[][])
    n602 = call-poly <vilib>:"DAQmx Write.vi"("task/channels in"=w1293, "auto start"=TRUE, "data"=w1288, "error in"=w1292) -> ("task out"=w1295:refnum<k21>, "error out"=w1296:errorcluster)  [unwired: 9 in, 1 out]
    n603 = call-poly <vilib>:"DAQmx Write.vi"("task/channels in"=w1275, "auto start"=TRUE, "data"=w1270, "error in"=w1274) -> ("task out"=w1277:refnum<k21>, "error out"=w1278:errorcluster)  [unwired: 9 in, 1 out]
    n604 = call <vilib>:"DAQmx Clear Task.vi"("task in"=w1295, "error in"=w1296) -> ("error out"=w1290:errorcluster)  [unwired: 13 in]
    n605 = call <vilib>:"DAQmx Clear Task.vi"("task in"=w1277, "error in"=w1278) -> ("error out"=w1272:errorcluster)  [unwired: 13 in]
    n606 = call <vilib>:"Simple Error Handler.vi"("error in (no error)"=w1290) -> ()  [unwired: 4 in, 5 out]
    n607 = call <vilib>:"Simple Error Handler.vi"("error in (no error)"=w1272) -> ()  [unwired: 4 in, 5 out]
  }
  n608 = while {
    shift-left: 0.0 ("Plant Output") -> [w1425]
    shift-right: [w1420] -> _
    tunnel: w37 -> [_]
    shift-right: [w1406] -> _
    shift-left: 0.01 -> [w1404]
    shift-right: [w1378] -> _
    shift-left: TRUE -> [w1403]
    shift-right: [w1380] -> _
    shift-left: w34 -> [w1402]
    shift-right: [w1405] -> _
    shift-left: w34 -> [w1401]
    tunnel: [w1375] -> w33
    tunnel: w14 -> [w1361]
    tunnel: [w1360] -> w3
    stop <- "Stop 9" stop-if-true
    w1366 = 1 items=["one channel for each line", "one channel for all lines"] ("line grouping")
    w1375 = 0.05 ("Sampling Time dt (s)")
    w1384 = 1 items=["one channel for each line", "one channel for all lines"] ("line grouping")
    w1392 = 0.5 ("x")
    w1419 = T7 {"static gain"=2.5, "lag (s)"=2.5, "deadtime (s)"=0.01, "load"=0.0, "deadband"=0.0, "sensor noise"=0.0, "initial PV"=30.0, "plant noise"=0.0}  # Process parameters
    w1421 = FALSE  # Integrator ?
    # "C."
    # "Inlet 11"
    # "Exhaust 4"
    # "B."
    # "A."
    # "A.Output to PWM Logic \nB. Simulated Plant\nC. Draw Chart"
    # "Main PID Loop Control"
    n609 = Multiply(x=w1375, y=1000.0) -> (x*y=w1418:dbl)
    n610 = Not(x="Autotune 9") -> (.not. x?=w1422:bool)
    n611 = feedback #25() -> (w1427:bool)  [unwired: 1 in]
    n612 = feedback-in #25("Autotune 9") -> ()
    n613 = Wait Until Next ms Multiple(millisecond multiple=w1418) -> ()  [unwired: 1 out]
    n614 = Exclusive Or(1:w1427, 2:"Autotune 9") -> (0:w1426:bool)
    n615 = feedback #26() -> (w1424:dbl)  [unwired: 1 in]
    n616 = Multiply(x=w1361, y=-1000.0) -> (x*y=w1408:dynamicdata)
    n617 = call <vilib>:"Median PtByPt.vi"("sample length"="Median sample length 18", "x"=w1408) -> ("median"=w1407:dbl)  [unwired: 2 in, 1 out]
    n618 = Square(x=w1407) -> (x^2=w1415:dbl)
    n619 = Multiply(x=w1407, y=-39.646) -> (x*y=w1411:dbl)
    n620 = Multiply(x=w1415, y=0.2324) -> (x*y=w1412:dbl)
    n621 = Add(x=w1411, y=w1412) -> (x+y=w1410:dbl)
    n622 = Add(x=1678.0, y=w1410) -> (x+y=w1373:dbl)
    n623 = case shown="False" "Autotune 9" {
      tunnel: w1375 -> [w1442 _]
      tunnel: [w1431 w1447] -> w1380
      tunnel: w1425 -> [_ w1446]
      tunnel: "PID Gains 9" -> [w1441 _]
      tunnel: "Reinitialize 9" -> [w1438 _]
      tunnel: w1426 -> [w1440 w1445]
      tunnel: w1424 -> [_ w1449]
      tunnel: w1373 -> [w1434 _]
      tunnel: "Set Point 9" -> [w1433 _]
      frame False {
        # "This code is to have 'bumpless' transfer from autotuning"
        n624 = Not(x=w1440) -> (.not. x?=w1437:bool)
        n625 = And(x="Automatic 9", y=w1437) -> (x .and. y?=w1439:bool)
        n626 = call-poly <vilib>:"PID Advanced.vi"("setpoint"=w1433, "auto? (T)"=w1439, "manual control"="MV: 9", "process variable"=w1434, "alpha"=10.0, "PID gains"=w1441, "dt (s)"=w1442, "reinitialize? (F)"=w1438) -> ("output"=w1431:dbl)  [unwired: 6 in, 1 out]
      }
      frame True {
        w1452 = 10000 ("sample length")
        # "Buffering data for parameters estimation"
        n627 = call <vilib>:"Data Queue PtByPt.vi"("initial queue element"=w1446, "initialize"=w1445, "sample length"=w1452, "input data point"=w1446) -> ("Current Queue"=→"Control Output 9":dbl[])  [unwired: 3 in, 4 out]
        n628 = Select(t=0.0, s=w1445, f="Excitation 9") -> (s? t:f=w1450:dbl)
        n629 = Add(x=w1449, y=w1450) -> (x+y=w1447:dbl)
        n630 = call <vilib>:"Data Queue PtByPt.vi"("initial queue element"=w1447, "initialize"=w1445, "sample length"=w1452, "input data point"=w1447) -> ("Current Queue"=→"Measurement 9":dbl[])  [unwired: 3 in, 4 out]
      }
    }
    n631 = feedback-in #26(w1380, w1422) -> ()
    n632 = Greater?(x=w1373, y="M-4") -> (0:w1360:bool)
    n633 = Add(x=w1404, y=w1392) -> (x+y=w1393:dbl)
    n634 = Subtract(x=w1404, y=w1392) -> (x-y=w1391:dbl)
    n635 = Equal?(x=w1402, y=w1380) -> (x = y?=w1399:bool)
    n636 = Greater?(x=w1380, y=w1402) -> (0:w1398:bool)
    n637 = Select(t=w1403, s=w1399, f=w1398) -> (s? t:f=w1378:bool)
    "PWM Output 9" <- w1378
    n638 = call "Plant System.vi"("Integrator ?"=w1421, "Plant Input"=w1380, "dt (s)"=w1375, "process parameters"=w1419) -> ("Plant Output"=w1420:dbl)  [unwired: 11 in]
    n639 = Increment(x="Set Point 9") -> (x+1=w1397:dbl)
    n640 = Decrement(x="Set Point 9") -> (x-1=w1396:dbl)
    n641 = Select(t=w1393, s=w1378, f=w1391) -> (s? t:f=w1406:dbl)
    n642 = Select(t=w1397, s=w1378, f=w1396) -> (s? t:f=w1395:dbl)
    n643 = Not(x=w1378) -> (.not. x?=w1377:bool)
    n644 = call-poly <vilib>:"DAQmx Create Virtual Channel.vi"("lines"=tag "cDAQ1Mod8/port0/line5", "line grouping"=w1384) -> ("task out"=w1386:refnum<k21>, "error out"=w1385:errorcluster)  [unwired: 12 in]
    n645 = call-poly <vilib>:"DAQmx Create Virtual Channel.vi"("lines"=tag "cDAQ1Mod7/port0/line4", "line grouping"=w1366) -> ("task out"=w1368:refnum<k21>, "error out"=w1367:errorcluster)  [unwired: 12 in]
    n646 = Build Array(w1373, "Set Point 9", w1395) -> (w1394:dbl[])
    n647 = Initialize Array("INLET 10 ON/OFF 2", 1 ("dimension size")) -> (w1363:bool[])
    n648 = Initialize Array(w1377, 1 ("dimension size")) -> (w1381:bool[])
    n649 = local write "MV: 9"(w1380) -> ()
    n650 = Add(x=w1401, y=w1404) -> (x+y=w1405:dbl)
    n651 = Build Array(w1394) -> (→"Real time Data 9":dbl[][])
    n652 = call-poly <vilib>:"DAQmx Write.vi"("task/channels in"=w1386, "auto start"=TRUE, "data"=w1381, "error in"=w1385) -> ("task out"=w1388:refnum<k21>, "error out"=w1389:errorcluster)  [unwired: 9 in, 1 out]
    n653 = call-poly <vilib>:"DAQmx Write.vi"("task/channels in"=w1368, "auto start"=TRUE, "data"=w1363, "error in"=w1367) -> ("task out"=w1370:refnum<k21>, "error out"=w1371:errorcluster)  [unwired: 9 in, 1 out]
    n654 = call <vilib>:"DAQmx Clear Task.vi"("task in"=w1388, "error in"=w1389) -> ("error out"=w1383:errorcluster)  [unwired: 13 in]
    n655 = call <vilib>:"DAQmx Clear Task.vi"("task in"=w1370, "error in"=w1371) -> ("error out"=w1365:errorcluster)  [unwired: 13 in]
    n656 = call <vilib>:"Simple Error Handler.vi"("error in (no error)"=w1383) -> ()  [unwired: 4 in, 5 out]
    n657 = call <vilib>:"Simple Error Handler.vi"("error in (no error)"=w1365) -> ()  [unwired: 4 in, 5 out]
  }
  n658 = while {
    shift-left: 0.0 ("Plant Output") -> [w1518]
    shift-right: [w1513] -> _
    tunnel: w43 -> [_]
    shift-right: [w1499] -> _
    shift-left: 0.01 -> [w1497]
    shift-right: [w1471] -> _
    shift-left: TRUE -> [w1496]
    shift-right: [w1473] -> _
    shift-left: w40 -> [w1495]
    shift-right: [w1498] -> _
    shift-left: w40 -> [w1494]
    tunnel: [w1468] -> w39
    tunnel: w14 -> [w1454]
    tunnel: [w1453] -> w2
    stop <- "Stop 8" stop-if-true
    w1459 = 1 items=["one channel for each line", "one channel for all lines"] ("line grouping")
    w1468 = 0.05 ("Sampling Time dt (s)")
    w1477 = 1 items=["one channel for each line", "one channel for all lines"] ("line grouping")
    w1485 = 0.5 ("x")
    w1512 = T7 {"static gain"=2.5, "lag (s)"=2.5, "deadtime (s)"=0.01, "load"=0.0, "deadband"=0.0, "sensor noise"=0.0, "initial PV"=30.0, "plant noise"=0.0}  # Process parameters
    w1514 = FALSE  # Integrator ?
    # "C."
    # "Inlet 11"
    # "Exhaust 2"
    # "B."
    # "A."
    # "A.Output to PWM Logic \nB. Simulated Plant\nC. Draw Chart"
    # "Main PID Loop Control"
    n659 = Multiply(x=w1468, y=1000.0) -> (x*y=w1511:dbl)
    n660 = Not(x="Autotune 8") -> (.not. x?=w1515:bool)
    n661 = feedback #27() -> (w1520:bool)  [unwired: 1 in]
    n662 = feedback-in #27("Autotune 8") -> ()
    n663 = Wait Until Next ms Multiple(millisecond multiple=w1511) -> ()  [unwired: 1 out]
    n664 = Exclusive Or(1:w1520, 2:"Autotune 8") -> (0:w1519:bool)
    n665 = feedback #28() -> (w1517:dbl)  [unwired: 1 in]
    n666 = Multiply(x=w1454, y=-1000.0) -> (x*y=w1501:dynamicdata)
    n667 = call <vilib>:"Median PtByPt.vi"("sample length"="Median sample length 17", "x"=w1501) -> ("median"=w1500:dbl)  [unwired: 2 in, 1 out]
    n668 = Square(x=w1500) -> (x^2=w1508:dbl)
    n669 = Multiply(x=w1500, y=-39.646) -> (x*y=w1504:dbl)
    n670 = Multiply(x=w1508, y=0.2324) -> (x*y=w1505:dbl)
    n671 = Add(x=w1504, y=w1505) -> (x+y=w1503:dbl)
    n672 = Add(x=1678.0, y=w1503) -> (x+y=w1466:dbl)
    n673 = case shown="False" "Autotune 8" {
      tunnel: w1468 -> [w1535 _]
      tunnel: [w1524 w1540] -> w1473
      tunnel: w1518 -> [_ w1539]
      tunnel: "PID Gains 8" -> [w1534 _]
      tunnel: "Reinitialize 8" -> [w1531 _]
      tunnel: w1519 -> [w1533 w1538]
      tunnel: w1517 -> [_ w1542]
      tunnel: w1466 -> [w1527 _]
      tunnel: "Set Point 8" -> [w1526 _]
      frame False {
        # "This code is to have 'bumpless' transfer from autotuning"
        n674 = Not(x=w1533) -> (.not. x?=w1530:bool)
        n675 = And(x="Automatic 8", y=w1530) -> (x .and. y?=w1532:bool)
        n676 = call-poly <vilib>:"PID Advanced.vi"("setpoint"=w1526, "auto? (T)"=w1532, "manual control"="MV: 8", "process variable"=w1527, "alpha"=10.0, "PID gains"=w1534, "dt (s)"=w1535, "reinitialize? (F)"=w1531) -> ("output"=w1524:dbl)  [unwired: 6 in, 1 out]
      }
      frame True {
        w1545 = 10000 ("sample length")
        # "Buffering data for parameters estimation"
        n677 = call <vilib>:"Data Queue PtByPt.vi"("initial queue element"=w1539, "initialize"=w1538, "sample length"=w1545, "input data point"=w1539) -> ("Current Queue"=→"Control Output 8":dbl[])  [unwired: 3 in, 4 out]
        n678 = Select(t=0.0, s=w1538, f="Excitation 8") -> (s? t:f=w1543:dbl)
        n679 = Add(x=w1542, y=w1543) -> (x+y=w1540:dbl)
        n680 = call <vilib>:"Data Queue PtByPt.vi"("initial queue element"=w1540, "initialize"=w1538, "sample length"=w1545, "input data point"=w1540) -> ("Current Queue"=→"Measurement 8":dbl[])  [unwired: 3 in, 4 out]
      }
    }
    n681 = feedback-in #28(w1473, w1515) -> ()
    n682 = Greater?(x=w1466, y="M-2") -> (0:w1453:bool)
    n683 = Add(x=w1497, y=w1485) -> (x+y=w1486:dbl)
    n684 = Subtract(x=w1497, y=w1485) -> (x-y=w1484:dbl)
    n685 = Equal?(x=w1495, y=w1473) -> (x = y?=w1492:bool)
    n686 = Greater?(x=w1473, y=w1495) -> (0:w1491:bool)
    n687 = Select(t=w1496, s=w1492, f=w1491) -> (s? t:f=w1471:bool)
    "PWM Output 8" <- w1471
    n688 = call "Plant System.vi"("Integrator ?"=w1514, "Plant Input"=w1473, "dt (s)"=w1468, "process parameters"=w1512) -> ("Plant Output"=w1513:dbl)  [unwired: 11 in]
    n689 = Increment(x="Set Point 8") -> (x+1=w1490:dbl)
    n690 = Decrement(x="Set Point 8") -> (x-1=w1489:dbl)
    n691 = Select(t=w1486, s=w1471, f=w1484) -> (s? t:f=w1499:dbl)
    n692 = Select(t=w1490, s=w1471, f=w1489) -> (s? t:f=w1488:dbl)
    n693 = Not(x=w1471) -> (.not. x?=w1470:bool)
    n694 = call-poly <vilib>:"DAQmx Create Virtual Channel.vi"("lines"=tag "cDAQ1Mod1/port0/line6", "line grouping"=w1477) -> ("task out"=w1479:refnum<k21>, "error out"=w1478:errorcluster)  [unwired: 12 in]
    n695 = call-poly <vilib>:"DAQmx Create Virtual Channel.vi"("lines"=tag "cDAQ1Mod2/port0/line6", "line grouping"=w1459) -> ("task out"=w1461:refnum<k21>, "error out"=w1460:errorcluster)  [unwired: 12 in]
    n696 = Build Array(w1466, "Set Point 8", w1488) -> (w1487:dbl[])
    n697 = Initialize Array("INLET 2 ON/OFF 2", 1 ("dimension size")) -> (w1456:bool[])
    n698 = Initialize Array(w1470, 1 ("dimension size")) -> (w1474:bool[])
    n699 = local write "MV: 8"(w1473) -> ()
    n700 = Add(x=w1494, y=w1497) -> (x+y=w1498:dbl)
    n701 = Build Array(w1487) -> (→"Real time Data 8":dbl[][])
    n702 = call-poly <vilib>:"DAQmx Write.vi"("task/channels in"=w1479, "auto start"=TRUE, "data"=w1474, "error in"=w1478) -> ("task out"=w1481:refnum<k21>, "error out"=w1482:errorcluster)  [unwired: 9 in, 1 out]
    n703 = call-poly <vilib>:"DAQmx Write.vi"("task/channels in"=w1461, "auto start"=TRUE, "data"=w1456, "error in"=w1460) -> ("task out"=w1463:refnum<k21>, "error out"=w1464:errorcluster)  [unwired: 9 in, 1 out]
    n704 = call <vilib>:"DAQmx Clear Task.vi"("task in"=w1481, "error in"=w1482) -> ("error out"=w1476:errorcluster)  [unwired: 13 in]
    n705 = call <vilib>:"DAQmx Clear Task.vi"("task in"=w1463, "error in"=w1464) -> ("error out"=w1458:errorcluster)  [unwired: 13 in]
    n706 = call <vilib>:"Simple Error Handler.vi"("error in (no error)"=w1476) -> ()  [unwired: 4 in, 5 out]
    n707 = call <vilib>:"Simple Error Handler.vi"("error in (no error)"=w1458) -> ()  [unwired: 4 in, 5 out]
  }
  n708 = while {
    shift-left: 0.0 ("Plant Output") -> [w1611]
    shift-right: [w1606] -> _
    tunnel: w49 -> [_]
    shift-right: [w1592] -> _
    shift-left: 0.01 -> [w1590]
    shift-right: [w1564] -> _
    shift-left: TRUE -> [w1589]
    shift-right: [w1566] -> _
    shift-left: w46 -> [w1588]
    shift-right: [w1591] -> _
    shift-left: w46 -> [w1587]
    tunnel: [w1561] -> w45
    tunnel: w14 -> [w1547]
    tunnel: [w1546] -> w1
    stop <- "Stop 7" stop-if-true
    w1552 = 1 items=["one channel for each line", "one channel for all lines"] ("line grouping")
    w1561 = 0.05 ("Sampling Time dt (s)")
    w1570 = 1 items=["one channel for each line", "one channel for all lines"] ("line grouping")
    w1578 = 0.5 ("x")
    w1605 = T7 {"static gain"=2.5, "lag (s)"=2.5, "deadtime (s)"=0.01, "load"=0.0, "deadband"=0.0, "sensor noise"=0.0, "initial PV"=30.0, "plant noise"=0.0}  # Process parameters
    w1607 = FALSE  # Integrator ?
    # "C."
    # "Inlet 11"
    # "Exhaust 7"
    # "B."
    # "A."
    # "A.Output to PWM Logic \nB. Simulated Plant\nC. Draw Chart"
    # "Main PID Loop Control"
    n709 = Multiply(x=w1561, y=1000.0) -> (x*y=w1604:dbl)
    n710 = Not(x="Autotune 7") -> (.not. x?=w1608:bool)
    n711 = feedback #29() -> (w1613:bool)  [unwired: 1 in]
    n712 = feedback-in #29("Autotune 7") -> ()
    n713 = Wait Until Next ms Multiple(millisecond multiple=w1604) -> ()  [unwired: 1 out]
    n714 = Exclusive Or(1:w1613, 2:"Autotune 7") -> (0:w1612:bool)
    n715 = feedback #30() -> (w1610:dbl)  [unwired: 1 in]
    n716 = Multiply(x=w1547, y=-1000.0) -> (x*y=w1594:dynamicdata)
    n717 = call <vilib>:"Median PtByPt.vi"("sample length"="Median sample length 16", "x"=w1594) -> ("median"=w1593:dbl)  [unwired: 2 in, 1 out]
    n718 = Square(x=w1593) -> (x^2=w1601:dbl)
    n719 = Multiply(x=w1593, y=-39.646) -> (x*y=w1597:dbl)
    n720 = Multiply(x=w1601, y=0.2324) -> (x*y=w1598:dbl)
    n721 = Add(x=w1597, y=w1598) -> (x+y=w1596:dbl)
    n722 = Add(x=1678.0, y=w1596) -> (x+y=w1559:dbl)
    n723 = case shown="False" "Autotune 7" {
      tunnel: w1561 -> [w1628 _]
      tunnel: [w1617 w1633] -> w1566
      tunnel: w1611 -> [_ w1632]
      tunnel: "PID Gains 7" -> [w1627 _]
      tunnel: "Reinitialize 7" -> [w1624 _]
      tunnel: w1612 -> [w1626 w1631]
      tunnel: w1610 -> [_ w1635]
      tunnel: w1559 -> [w1620 _]
      tunnel: "Set Point 7" -> [w1619 _]
      frame False {
        # "This code is to have 'bumpless' transfer from autotuning"
        n724 = Not(x=w1626) -> (.not. x?=w1623:bool)
        n725 = And(x="Automatic 7", y=w1623) -> (x .and. y?=w1625:bool)
        n726 = call-poly <vilib>:"PID Advanced.vi"("setpoint"=w1619, "auto? (T)"=w1625, "manual control"="MV: 7", "process variable"=w1620, "alpha"=10.0, "PID gains"=w1627, "dt (s)"=w1628, "reinitialize? (F)"=w1624) -> ("output"=w1617:dbl)  [unwired: 6 in, 1 out]
      }
      frame True {
        w1638 = 10000 ("sample length")
        # "Buffering data for parameters estimation"
        n727 = call <vilib>:"Data Queue PtByPt.vi"("initial queue element"=w1632, "initialize"=w1631, "sample length"=w1638, "input data point"=w1632) -> ("Current Queue"=→"Control Output 7":dbl[])  [unwired: 3 in, 4 out]
        n728 = Select(t=0.0, s=w1631, f="Excitation 7") -> (s? t:f=w1636:dbl)
        n729 = Add(x=w1635, y=w1636) -> (x+y=w1633:dbl)
        n730 = call <vilib>:"Data Queue PtByPt.vi"("initial queue element"=w1633, "initialize"=w1631, "sample length"=w1638, "input data point"=w1633) -> ("Current Queue"=→"Measurement 7":dbl[])  [unwired: 3 in, 4 out]
      }
    }
    n731 = feedback-in #30(w1566, w1608) -> ()
    n732 = Greater?(x=w1559, y="M-7") -> (0:w1546:bool)
    n733 = Add(x=w1590, y=w1578) -> (x+y=w1579:dbl)
    n734 = Subtract(x=w1590, y=w1578) -> (x-y=w1577:dbl)
    n735 = Equal?(x=w1588, y=w1566) -> (x = y?=w1585:bool)
    n736 = Greater?(x=w1566, y=w1588) -> (0:w1584:bool)
    n737 = Select(t=w1589, s=w1585, f=w1584) -> (s? t:f=w1564:bool)
    "PWM Output 7" <- w1564
    n738 = call "Plant System.vi"("Integrator ?"=w1607, "Plant Input"=w1566, "dt (s)"=w1561, "process parameters"=w1605) -> ("Plant Output"=w1606:dbl)  [unwired: 11 in]
    n739 = Increment(x="Set Point 7") -> (x+1=w1583:dbl)
    n740 = Decrement(x="Set Point 7") -> (x-1=w1582:dbl)
    n741 = Select(t=w1579, s=w1564, f=w1577) -> (s? t:f=w1592:dbl)
    n742 = Select(t=w1583, s=w1564, f=w1582) -> (s? t:f=w1581:dbl)
    n743 = Not(x=w1564) -> (.not. x?=w1563:bool)
    n744 = call-poly <vilib>:"DAQmx Create Virtual Channel.vi"("lines"=tag "cDAQ1Mod8/port0/line4", "line grouping"=w1570) -> ("task out"=w1572:refnum<k21>, "error out"=w1571:errorcluster)  [unwired: 12 in]
    n745 = call-poly <vilib>:"DAQmx Create Virtual Channel.vi"("lines"=tag "cDAQ1Mod7/port0/line3", "line grouping"=w1552) -> ("task out"=w1554:refnum<k21>, "error out"=w1553:errorcluster)  [unwired: 12 in]
    n746 = Build Array(w1559, "Set Point 7", w1581) -> (w1580:dbl[])
    n747 = Initialize Array("INLET 7 ON/OFF 2", 1 ("dimension size")) -> (w1549:bool[])
    n748 = Initialize Array(w1563, 1 ("dimension size")) -> (w1567:bool[])
    n749 = local write "MV: 7"(w1566) -> ()
    n750 = Add(x=w1587, y=w1590) -> (x+y=w1591:dbl)
    n751 = Build Array(w1580) -> (→"Real time Data 7":dbl[][])
    n752 = call-poly <vilib>:"DAQmx Write.vi"("task/channels in"=w1572, "auto start"=TRUE, "data"=w1567, "error in"=w1571) -> ("task out"=w1574:refnum<k21>, "error out"=w1575:errorcluster)  [unwired: 9 in, 1 out]
    n753 = call-poly <vilib>:"DAQmx Write.vi"("task/channels in"=w1554, "auto start"=TRUE, "data"=w1549, "error in"=w1553) -> ("task out"=w1556:refnum<k21>, "error out"=w1557:errorcluster)  [unwired: 9 in, 1 out]
    n754 = call <vilib>:"DAQmx Clear Task.vi"("task in"=w1574, "error in"=w1575) -> ("error out"=w1569:errorcluster)  [unwired: 13 in]
    n755 = call <vilib>:"DAQmx Clear Task.vi"("task in"=w1556, "error in"=w1557) -> ("error out"=w1551:errorcluster)  [unwired: 13 in]
    n756 = call <vilib>:"Simple Error Handler.vi"("error in (no error)"=w1569) -> ()  [unwired: 4 in, 5 out]
    n757 = call <vilib>:"Simple Error Handler.vi"("error in (no error)"=w1551) -> ()  [unwired: 4 in, 5 out]
  }
  n758 = Compound Arithmetic op=OR(w11, w13, w10, w9, w8, w7, w6, w5, w4, w3, w2, w1) -> (w12:bool)
  "?" <- w12
  n759 = case shown="True" w12 {
    frame False {
    }
    frame True {
      n760 = call <vilib>:"Beep.vi"("use system alert? (T)"=FALSE, "duration (msec)"=u32 2000, "frequency (Hz)"=u32 15000) -> ()  [unwired: 9 in]
    }
  }
  n761 = control-ref of="stop"() -> (w100:refnum<vi>)
  n762 = control-ref of="XYZAER"() -> (w91:refnum<vi>)
  n763 = control-ref of="PnoData"() -> (w82:refnum<vi>)
  n764 = call <instrlib>:"PDI data xyzaer loop.vi"("Data Ready Refnum"=w82, "FrameCount Ctl Ref"=w92, "error in (no error)"=w102, "xyzaer array\nRefnum"=w91, "Stop Ctl Ref"=w100, "pDev"=w101) -> ("error out"=w89:errorcluster, "Loop Iter"=w93:i32, "dup pDev"=w90:u32)  [unwired: 3 out]
  n765 = local write "Loop Iter"(w93) -> ()
  n766 = local write "Stop 11"(w25) -> ()
  n767 = local write "Stop 12"(w19) -> ()
  n768 = local write "Stop 10"(w31) -> ()
  n769 = local write "Stop 9"(w37) -> ()
  n770 = call <instrlib>:"PDI action stopcont.vi"("error in (no error)"=w89, "pDev"=w90) -> ("error out"=w98:errorcluster, "Running"=w103:bool, "dup pDev"=w104:u32)  [unwired: 7 out]
  n771 = local write "Stop 8"(w43) -> ()
  n772 = local write "Stop 7"(w49) -> ()
  n773 = local write "Running"(w103) -> ()
  n774 = case shown="No Error" w89 {
    tunnel: w97 -> [w1642 _]
    frame No Error {
      # "Success up to here"
      n775 = call "Elapsed Time"("Set Start Time (s)"=w1642) -> ("Present Text"=w1644:string, "Elapsed Time Text"=w1643:string)  [unwired: 4 in, 13 out]
      n776 = local write "Stop Time Text"(w1644) -> ()
      n777 = local write "Elapsed Time Text"(w1643) -> ()
    }
    frame Error {
      # "Error somewhere;\nStop Time is irrelevant"
    }
  }
  n778 = while {
    tunnel: w25 -> [_]
    tunnel: w21 -> [w1648]
    stop <- w1658 stop-if-true
    # "If dT and deadtime have similar values, the identification could evaluate deadtime as zero and this generates proportional gain equal to Inf. This code avoid gain changes in this situations."
    # "Autotuning Loop"
    n779 = local read "Control Output 11"() -> (w1660:dbl[])
    n780 = local read "Measurement 11"() -> (w1659:dbl[])
    n781 = case shown="\"Chien-Hrones-Reswick\"" "Control 11" {
      tunnel: w1660 -> [w1669 w1677 w1686 w1695]
      tunnel: w1659 -> [w1668 w1676 w1685 w1694]
      tunnel: [w1667 w1675 w1684 w1693] -> w1647
      tunnel: [w1666 w1674 w1683 w1692] -> w1646
      tunnel: w1648 -> [w1665 w1673 w1682 w1691]
      tunnel: [w1664 w1672 w1681 w1690] -> w1645
      tunnel: [w1663 w1671 w1680 w1689] -> w1650
      tunnel: "Type of controller 11" -> [w1662 w1670 w1679 w1688]
      frame "Ziegler-Nichols", Default {
        n782 = call-poly <vilib>:"PID Autotuning Design.vi"("Ziegler-Nichols Speed"="Ziegler-Nichols speed 11", "Type of Controller"=w1662, "dt (s)"=w1665, "Response signal"=w1668, "Stimulus signal"=w1669) -> ("PID gains"=w1663:T2, "response operating point"=w1666:dbl, "stimulus operating point"=w1667:dbl, "Plant Parameters"=w1664:T4)  [unwired: 3 in]
      }
      frame "Cohen-Coon" {
        n783 = call-poly <vilib>:"PID Autotuning Design.vi"("Type of Controller"=w1670, "dt (s)"=w1673, "Response signal"=w1676, "Stimulus signal"=w1677) -> ("PID gains"=w1671:T2, "response offset"=w1674:dbl, "stimulus offset"=w1675:dbl, "Plant Parameters"=w1672:T4)  [unwired: 4 in]
      }
      frame "Chien-Hrones-Reswick" {
        n784 = call-poly <vilib>:"PID Autotuning Design.vi"("Tuning specifications"="Tuning specifications 11", "Type of Controller"=w1679, "dt (s)"=w1682, "Response signal"=w1685, "Stimulus signal"=w1686) -> ("PID gains"=w1680:T2, "response offset"=w1683:dbl, "stimulus offset"=w1684:dbl, "Plant Parameters"=w1681:T4)  [unwired: 3 in]
      }
      frame "Internal Model Control" {
        n785 = call-poly <vilib>:"PID Autotuning Design.vi"("Desired Time Constant (tau_c)"="Multiplicative factor 11", "Type of Controller"=w1688, "dt (s)"=w1691, "Response signal"=w1694, "Stimulus signal"=w1695) -> ("PID gains"=w1689:T2, "response offset"=w1692:dbl, "stimulus offset"=w1693:dbl, "Plant Parameters"=w1690:T4)  [unwired: 3 in]
      }
    }
    "Stimulus operating point 11" <- w1647
    "Response operating point 11" <- w1646
    "Identified Plant Parameters 11" <- w1645
    n786 = Unbundle(w1650) -> ("proportional gain (Kc)"=w1653:dbl)  [unwired: 2 out]
    n787 = Equal?(x=w1653, y=inf) -> (x = y?=w1652:bool)
    n788 = feedback #31() -> (w1651:T2)  [unwired: 1 in]
    n789 = Select(t=w1651, s=w1652, f=w1650) -> (s? t:f=w1649:T2)
    "Tuned PID gains 11" <- w1649
    n790 = feedback-in #31(w1649) -> ()
    n791 = case shown="True" "Accept gain 11" {
      tunnel: w1649 -> [_ w1696]
      frame False {
      }
      frame True {
        n792 = local write "PID Gains 11"(w1696) -> ()
      }
    }
    n793 = local read "Stop 11"() -> (w1658:bool)
  }
  n794 = while {
    tunnel: w19 -> [_]
    tunnel: w15 -> [w1700]
    stop <- w1710 stop-if-true
    # "If dT and deadtime have similar values, the identification could evaluate deadtime as zero and this generates proportional gain equal to Inf. This code avoid gain changes in this situations."
    # "Autotuning Loop"
    n795 = local read "Control Output 12"() -> (w1712:dbl[])
    n796 = local read "Measurement 12"() -> (w1711:dbl[])
    n797 = case shown="\"Chien-Hrones-Reswick\"" "Control 12" {
      tunnel: w1712 -> [w1721 w1729 w1738 w1747]
      tunnel: w1711 -> [w1720 w1728 w1737 w1746]
      tunnel: [w1719 w1727 w1736 w1745] -> w1699
      tunnel: [w1718 w1726 w1735 w1744] -> w1698
      tunnel: w1700 -> [w1717 w1725 w1734 w1743]
      tunnel: [w1716 w1724 w1733 w1742] -> w1697
      tunnel: [w1715 w1723 w1732 w1741] -> w1702
      tunnel: "Type of controller 12" -> [w1714 w1722 w1731 w1740]
      frame "Ziegler-Nichols", Default {
        n798 = call-poly <vilib>:"PID Autotuning Design.vi"("Ziegler-Nichols Speed"="Ziegler-Nichols speed 12", "Type of Controller"=w1714, "dt (s)"=w1717, "Response signal"=w1720, "Stimulus signal"=w1721) -> ("PID gains"=w1715:T2, "response operating point"=w1718:dbl, "stimulus operating point"=w1719:dbl, "Plant Parameters"=w1716:T4)  [unwired: 3 in]
      }
      frame "Cohen-Coon" {
        n799 = call-poly <vilib>:"PID Autotuning Design.vi"("Type of Controller"=w1722, "dt (s)"=w1725, "Response signal"=w1728, "Stimulus signal"=w1729) -> ("PID gains"=w1723:T2, "response offset"=w1726:dbl, "stimulus offset"=w1727:dbl, "Plant Parameters"=w1724:T4)  [unwired: 4 in]
      }
      frame "Chien-Hrones-Reswick" {
        n800 = call-poly <vilib>:"PID Autotuning Design.vi"("Tuning specifications"="Tuning specifications 12", "Type of Controller"=w1731, "dt (s)"=w1734, "Response signal"=w1737, "Stimulus signal"=w1738) -> ("PID gains"=w1732:T2, "response offset"=w1735:dbl, "stimulus offset"=w1736:dbl, "Plant Parameters"=w1733:T4)  [unwired: 3 in]
      }
      frame "Internal Model Control" {
        n801 = call-poly <vilib>:"PID Autotuning Design.vi"("Desired Time Constant (tau_c)"="Multiplicative factor 12", "Type of Controller"=w1740, "dt (s)"=w1743, "Response signal"=w1746, "Stimulus signal"=w1747) -> ("PID gains"=w1741:T2, "response offset"=w1744:dbl, "stimulus offset"=w1745:dbl, "Plant Parameters"=w1742:T4)  [unwired: 3 in]
      }
    }
    "Stimulus operating point 12" <- w1699
    "Response operating point 12" <- w1698
    "Identified Plant Parameters 12" <- w1697
    n802 = Unbundle(w1702) -> ("proportional gain (Kc)"=w1705:dbl)  [unwired: 2 out]
    n803 = Equal?(x=w1705, y=inf) -> (x = y?=w1704:bool)
    n804 = feedback #32() -> (w1703:T2)  [unwired: 1 in]
    n805 = Select(t=w1703, s=w1704, f=w1702) -> (s? t:f=w1701:T2)
    "Tuned PID gains 12" <- w1701
    n806 = feedback-in #32(w1701) -> ()
    n807 = case shown="True" "Accept gain 12" {
      tunnel: w1701 -> [_ w1748]
      frame False {
      }
      frame True {
        n808 = local write "PID Gains 12"(w1748) -> ()
      }
    }
    n809 = local read "Stop 12"() -> (w1710:bool)
  }
  n810 = while {
    tunnel: w31 -> [_]
    tunnel: w27 -> [w1752]
    stop <- w1762 stop-if-true
    # "If dT and deadtime have similar values, the identification could evaluate deadtime as zero and this generates proportional gain equal to Inf. This code avoid gain changes in this situations."
    # "Autotuning Loop"
    n811 = local read "Control Output 10"() -> (w1764:dbl[])
    n812 = local read "Measurement 10"() -> (w1763:dbl[])
    n813 = case shown="\"Chien-Hrones-Reswick\"" "Control 10" {
      tunnel: w1764 -> [w1773 w1781 w1790 w1799]
      tunnel: w1763 -> [w1772 w1780 w1789 w1798]
      tunnel: [w1771 w1779 w1788 w1797] -> w1751
      tunnel: [w1770 w1778 w1787 w1796] -> w1750
      tunnel: w1752 -> [w1769 w1777 w1786 w1795]
      tunnel: [w1768 w1776 w1785 w1794] -> w1749
      tunnel: [w1767 w1775 w1784 w1793] -> w1754
      tunnel: "Type of controller 10" -> [w1766 w1774 w1783 w1792]
      frame "Ziegler-Nichols", Default {
        n814 = call-poly <vilib>:"PID Autotuning Design.vi"("Ziegler-Nichols Speed"="Ziegler-Nichols speed 10", "Type of Controller"=w1766, "dt (s)"=w1769, "Response signal"=w1772, "Stimulus signal"=w1773) -> ("PID gains"=w1767:T2, "response operating point"=w1770:dbl, "stimulus operating point"=w1771:dbl, "Plant Parameters"=w1768:T4)  [unwired: 3 in]
      }
      frame "Cohen-Coon" {
        n815 = call-poly <vilib>:"PID Autotuning Design.vi"("Type of Controller"=w1774, "dt (s)"=w1777, "Response signal"=w1780, "Stimulus signal"=w1781) -> ("PID gains"=w1775:T2, "response offset"=w1778:dbl, "stimulus offset"=w1779:dbl, "Plant Parameters"=w1776:T4)  [unwired: 4 in]
      }
      frame "Chien-Hrones-Reswick" {
        n816 = call-poly <vilib>:"PID Autotuning Design.vi"("Tuning specifications"="Tuning specifications 10", "Type of Controller"=w1783, "dt (s)"=w1786, "Response signal"=w1789, "Stimulus signal"=w1790) -> ("PID gains"=w1784:T2, "response offset"=w1787:dbl, "stimulus offset"=w1788:dbl, "Plant Parameters"=w1785:T4)  [unwired: 3 in]
      }
      frame "Internal Model Control" {
        n817 = call-poly <vilib>:"PID Autotuning Design.vi"("Desired Time Constant (tau_c)"="Multiplicative factor 10", "Type of Controller"=w1792, "dt (s)"=w1795, "Response signal"=w1798, "Stimulus signal"=w1799) -> ("PID gains"=w1793:T2, "response offset"=w1796:dbl, "stimulus offset"=w1797:dbl, "Plant Parameters"=w1794:T4)  [unwired: 3 in]
      }
    }
    "Stimulus operating point 10" <- w1751
    "Response operating point 10" <- w1750
    "Identified Plant Parameters 10" <- w1749
    n818 = Unbundle(w1754) -> ("proportional gain (Kc)"=w1757:dbl)  [unwired: 2 out]
    n819 = Equal?(x=w1757, y=inf) -> (x = y?=w1756:bool)
    n820 = feedback #33() -> (w1755:T2)  [unwired: 1 in]
    n821 = Select(t=w1755, s=w1756, f=w1754) -> (s? t:f=w1753:T2)
    "Tuned PID gains 10" <- w1753
    n822 = feedback-in #33(w1753) -> ()
    n823 = case shown="True" "Accept gain 10" {
      tunnel: w1753 -> [_ w1800]
      frame False {
      }
      frame True {
        n824 = local write "PID Gains 10"(w1800) -> ()
      }
    }
    n825 = local read "Stop 10"() -> (w1762:bool)
  }
  n826 = while {
    tunnel: w37 -> [_]
    tunnel: w33 -> [w1804]
    stop <- w1814 stop-if-true
    # "If dT and deadtime have similar values, the identification could evaluate deadtime as zero and this generates proportional gain equal to Inf. This code avoid gain changes in this situations."
    # "Autotuning Loop"
    n827 = local read "Control Output 9"() -> (w1816:dbl[])
    n828 = local read "Measurement 9"() -> (w1815:dbl[])
    n829 = case shown="\"Chien-Hrones-Reswick\"" "Control 9" {
      tunnel: w1816 -> [w1825 w1833 w1842 w1851]
      tunnel: w1815 -> [w1824 w1832 w1841 w1850]
      tunnel: [w1823 w1831 w1840 w1849] -> w1803
      tunnel: [w1822 w1830 w1839 w1848] -> w1802
      tunnel: w1804 -> [w1821 w1829 w1838 w1847]
      tunnel: [w1820 w1828 w1837 w1846] -> w1801
      tunnel: [w1819 w1827 w1836 w1845] -> w1806
      tunnel: "Type of controller 9" -> [w1818 w1826 w1835 w1844]
      frame "Ziegler-Nichols", Default {
        n830 = call-poly <vilib>:"PID Autotuning Design.vi"("Ziegler-Nichols Speed"="Ziegler-Nichols speed 9", "Type of Controller"=w1818, "dt (s)"=w1821, "Response signal"=w1824, "Stimulus signal"=w1825) -> ("PID gains"=w1819:T2, "response operating point"=w1822:dbl, "stimulus operating point"=w1823:dbl, "Plant Parameters"=w1820:T4)  [unwired: 3 in]
      }
      frame "Cohen-Coon" {
        n831 = call-poly <vilib>:"PID Autotuning Design.vi"("Type of Controller"=w1826, "dt (s)"=w1829, "Response signal"=w1832, "Stimulus signal"=w1833) -> ("PID gains"=w1827:T2, "response offset"=w1830:dbl, "stimulus offset"=w1831:dbl, "Plant Parameters"=w1828:T4)  [unwired: 4 in]
      }
      frame "Chien-Hrones-Reswick" {
        n832 = call-poly <vilib>:"PID Autotuning Design.vi"("Tuning specifications"="Tuning specifications 9", "Type of Controller"=w1835, "dt (s)"=w1838, "Response signal"=w1841, "Stimulus signal"=w1842) -> ("PID gains"=w1836:T2, "response offset"=w1839:dbl, "stimulus offset"=w1840:dbl, "Plant Parameters"=w1837:T4)  [unwired: 3 in]
      }
      frame "Internal Model Control" {
        n833 = call-poly <vilib>:"PID Autotuning Design.vi"("Desired Time Constant (tau_c)"="Multiplicative factor 9", "Type of Controller"=w1844, "dt (s)"=w1847, "Response signal"=w1850, "Stimulus signal"=w1851) -> ("PID gains"=w1845:T2, "response offset"=w1848:dbl, "stimulus offset"=w1849:dbl, "Plant Parameters"=w1846:T4)  [unwired: 3 in]
      }
    }
    "Stimulus operating point 9" <- w1803
    "Response operating point 9" <- w1802
    "Identified Plant Parameters 9" <- w1801
    n834 = Unbundle(w1806) -> ("proportional gain (Kc)"=w1809:dbl)  [unwired: 2 out]
    n835 = Equal?(x=w1809, y=inf) -> (x = y?=w1808:bool)
    n836 = feedback #34() -> (w1807:T2)  [unwired: 1 in]
    n837 = Select(t=w1807, s=w1808, f=w1806) -> (s? t:f=w1805:T2)
    "Tuned PID gains 9" <- w1805
    n838 = feedback-in #34(w1805) -> ()
    n839 = case shown="True" "Accept gain 9" {
      tunnel: w1805 -> [_ w1852]
      frame False {
      }
      frame True {
        n840 = local write "PID Gains 9"(w1852) -> ()
      }
    }
    n841 = local read "Stop 9"() -> (w1814:bool)
  }
  n842 = while {
    tunnel: w43 -> [_]
    tunnel: w39 -> [w1856]
    stop <- w1866 stop-if-true
    # "If dT and deadtime have similar values, the identification could evaluate deadtime as zero and this generates proportional gain equal to Inf. This code avoid gain changes in this situations."
    # "Autotuning Loop"
    n843 = local read "Control Output 8"() -> (w1868:dbl[])
    n844 = local read "Measurement 8"() -> (w1867:dbl[])
    n845 = case shown="\"Chien-Hrones-Reswick\"" "Control 8" {
      tunnel: w1868 -> [w1877 w1885 w1894 w1903]
      tunnel: w1867 -> [w1876 w1884 w1893 w1902]
      tunnel: [w1875 w1883 w1892 w1901] -> w1855
      tunnel: [w1874 w1882 w1891 w1900] -> w1854
      tunnel: w1856 -> [w1873 w1881 w1890 w1899]
      tunnel: [w1872 w1880 w1889 w1898] -> w1853
      tunnel: [w1871 w1879 w1888 w1897] -> w1858
      tunnel: "Type of controller 8" -> [w1870 w1878 w1887 w1896]
      frame "Ziegler-Nichols", Default {
        n846 = call-poly <vilib>:"PID Autotuning Design.vi"("Ziegler-Nichols Speed"="Ziegler-Nichols speed 8", "Type of Controller"=w1870, "dt (s)"=w1873, "Response signal"=w1876, "Stimulus signal"=w1877) -> ("PID gains"=w1871:T2, "response operating point"=w1874:dbl, "stimulus operating point"=w1875:dbl, "Plant Parameters"=w1872:T4)  [unwired: 3 in]
      }
      frame "Cohen-Coon" {
        n847 = call-poly <vilib>:"PID Autotuning Design.vi"("Type of Controller"=w1878, "dt (s)"=w1881, "Response signal"=w1884, "Stimulus signal"=w1885) -> ("PID gains"=w1879:T2, "response offset"=w1882:dbl, "stimulus offset"=w1883:dbl, "Plant Parameters"=w1880:T4)  [unwired: 4 in]
      }
      frame "Chien-Hrones-Reswick" {
        n848 = call-poly <vilib>:"PID Autotuning Design.vi"("Tuning specifications"="Tuning specifications 8", "Type of Controller"=w1887, "dt (s)"=w1890, "Response signal"=w1893, "Stimulus signal"=w1894) -> ("PID gains"=w1888:T2, "response offset"=w1891:dbl, "stimulus offset"=w1892:dbl, "Plant Parameters"=w1889:T4)  [unwired: 3 in]
      }
      frame "Internal Model Control" {
        n849 = call-poly <vilib>:"PID Autotuning Design.vi"("Desired Time Constant (tau_c)"="Multiplicative factor 8", "Type of Controller"=w1896, "dt (s)"=w1899, "Response signal"=w1902, "Stimulus signal"=w1903) -> ("PID gains"=w1897:T2, "response offset"=w1900:dbl, "stimulus offset"=w1901:dbl, "Plant Parameters"=w1898:T4)  [unwired: 3 in]
      }
    }
    "Stimulus operating point 8" <- w1855
    "Response operating point 8" <- w1854
    "Identified Plant Parameters 8" <- w1853
    n850 = Unbundle(w1858) -> ("proportional gain (Kc)"=w1861:dbl)  [unwired: 2 out]
    n851 = Equal?(x=w1861, y=inf) -> (x = y?=w1860:bool)
    n852 = feedback #35() -> (w1859:T2)  [unwired: 1 in]
    n853 = Select(t=w1859, s=w1860, f=w1858) -> (s? t:f=w1857:T2)
    "Tuned PID gains 8" <- w1857
    n854 = feedback-in #35(w1857) -> ()
    n855 = case shown="True" "Accept gain 8" {
      tunnel: w1857 -> [_ w1904]
      frame False {
      }
      frame True {
        n856 = local write "PID Gains 8"(w1904) -> ()
      }
    }
    n857 = local read "Stop 8"() -> (w1866:bool)
  }
  n858 = while {
    tunnel: w49 -> [_]
    tunnel: w45 -> [w1908]
    stop <- w1918 stop-if-true
    # "If dT and deadtime have similar values, the identification could evaluate deadtime as zero and this generates proportional gain equal to Inf. This code avoid gain changes in this situations."
    # "Autotuning Loop"
    n859 = local read "Control Output 7"() -> (w1920:dbl[])
    n860 = local read "Measurement 7"() -> (w1919:dbl[])
    n861 = case shown="\"Chien-Hrones-Reswick\"" "Control 7" {
      tunnel: w1920 -> [w1929 w1937 w1946 w1955]
      tunnel: w1919 -> [w1928 w1936 w1945 w1954]
      tunnel: [w1927 w1935 w1944 w1953] -> w1907
      tunnel: [w1926 w1934 w1943 w1952] -> w1906
      tunnel: w1908 -> [w1925 w1933 w1942 w1951]
      tunnel: [w1924 w1932 w1941 w1950] -> w1905
      tunnel: [w1923 w1931 w1940 w1949] -> w1910
      tunnel: "Type of controller 7" -> [w1922 w1930 w1939 w1948]
      frame "Ziegler-Nichols", Default {
        n862 = call-poly <vilib>:"PID Autotuning Design.vi"("Ziegler-Nichols Speed"="Ziegler-Nichols speed 7", "Type of Controller"=w1922, "dt (s)"=w1925, "Response signal"=w1928, "Stimulus signal"=w1929) -> ("PID gains"=w1923:T2, "response operating point"=w1926:dbl, "stimulus operating point"=w1927:dbl, "Plant Parameters"=w1924:T4)  [unwired: 3 in]
      }
      frame "Cohen-Coon" {
        n863 = call-poly <vilib>:"PID Autotuning Design.vi"("Type of Controller"=w1930, "dt (s)"=w1933, "Response signal"=w1936, "Stimulus signal"=w1937) -> ("PID gains"=w1931:T2, "response offset"=w1934:dbl, "stimulus offset"=w1935:dbl, "Plant Parameters"=w1932:T4)  [unwired: 4 in]
      }
      frame "Chien-Hrones-Reswick" {
        n864 = call-poly <vilib>:"PID Autotuning Design.vi"("Tuning specifications"="Tuning specifications 7", "Type of Controller"=w1939, "dt (s)"=w1942, "Response signal"=w1945, "Stimulus signal"=w1946) -> ("PID gains"=w1940:T2, "response offset"=w1943:dbl, "stimulus offset"=w1944:dbl, "Plant Parameters"=w1941:T4)  [unwired: 3 in]
      }
      frame "Internal Model Control" {
        n865 = call-poly <vilib>:"PID Autotuning Design.vi"("Desired Time Constant (tau_c)"="Multiplicative factor 7", "Type of Controller"=w1948, "dt (s)"=w1951, "Response signal"=w1954, "Stimulus signal"=w1955) -> ("PID gains"=w1949:T2, "response offset"=w1952:dbl, "stimulus offset"=w1953:dbl, "Plant Parameters"=w1950:T4)  [unwired: 3 in]
      }
    }
    "Stimulus operating point 7" <- w1907
    "Response operating point 7" <- w1906
    "Identified Plant Parameters 7" <- w1905
    n866 = Unbundle(w1910) -> ("proportional gain (Kc)"=w1913:dbl)  [unwired: 2 out]
    n867 = Equal?(x=w1913, y=inf) -> (x = y?=w1912:bool)
    n868 = feedback #36() -> (w1911:T2)  [unwired: 1 in]
    n869 = Select(t=w1911, s=w1912, f=w1910) -> (s? t:f=w1909:T2)
    "Tuned PID gains 7" <- w1909
    n870 = feedback-in #36(w1909) -> ()
    n871 = case shown="True" "Accept gain 7" {
      tunnel: w1909 -> [_ w1956]
      frame False {
      }
      frame True {
        n872 = local write "PID Gains 7"(w1956) -> ()
      }
    }
    n873 = local read "Stop 7"() -> (w1918:bool)
  }
  n874 = call <instrlib>:"PDI close.vi"("error in (no error)"=w98, "pDev"=w104) -> ("error out"=→"error out":errorcluster, "connected"=w99:bool)  [unwired: 8 out]
  n875 = local write "Connected"(w99) -> ()
